vi "lv_icon.vi"(10 "Color icon in":T2, 11 "BW icon in":T2) -> (0 "Error code out":i32=43, 2 "Color icon out":T2, 3 "BW icon out":T2)   [LabVIEW 2021, in "lv_icon.lvlib"]
doc: "<p>Display this dialog box in one of the following ways:</p>\n\n<ul>\n<li>Double-click the <a href=\"nihelplauncher://docs/csh?context=lvcore_lvconcepts_using_icons\">icon</a> in the upper right corner of the front panel window, block diagram window, or <a href=\"nihelplauncher://docs/csh?context=lvcore_lvconcepts_custom_cont_ind_type\">Control Editor</a> window.</li>\n<li>Right-click the icon in the upper right corner of the front panel window, block diagram window, or <strong>Control Editor</strong> window and select <strong>Edit Icon</strong> from the shortcut menu.</li>\n<li>Select <strong>File<span class=\"U+187\">>></span>VI Properties</strong> or <strong>File<span class=\"U+187\">>></span>Control Properties</strong> to display the <a href=\"nihelplauncher://docs/csh?context=lvcore_lvdialog_vi_properties_dialog_box\">VI Properties</a> dialog box or <strong>Control Properties</strong> dialog box, respectively. Then select <strong>General</strong> from the <strong>Category</strong> pull-down menu and click the <strong>Edit Icon</strong> button.</li>\n<li>Right-click a project library, statechart, class, or XControl item in the <a href=\"nihelplauncher://docs/csh?context=lvcore_lvconcepts_using_labview_projects\">Project Explorer</a> window and select <strong> Properties</strong> from the shortcut menu to display the corresponding <strong>Properties</strong> dialog box. Then click the <strong>Edit</strong> button on the <strong>General Settings</strong> page.</li>\n</ul>\n\n<p>Use this dialog box to <a href=\"nihelplauncher://docs/csh?context=lvcore_lvhowto_creating_icons\">create and edit icons</a>.</p>"
uses:
  <vilib>/LabVIEW Icon API/lv_icon/lv_icon.lvlib
  <vilib>/LabVIEW Icon API/lv_icon/Controls/BodyText.ctl
  <vilib>/LabVIEW Icon API/lv_icon/Controls/Font.ctl
  <vilib>/LabVIEW Icon API/lv_icon/Controls/Alignment.ctl
  <vilib>/LabVIEW Icon API/lv_icon/Controls/Layer.ctl
  <resource>/plugins/NIIconEditor/Controls/LayerList.ctl
  <resource>/plugins/NIIconEditor/Controls/NewLayer.ctl
  <resource>/plugins/NIIconEditor/Controls/DeleteLayer.ctl
  <resource>/plugins/NIIconEditor/Controls/Arrow Up.ctl
  <resource>/plugins/NIIconEditor/Controls/Arrow Down.ctl
  <resource>/plugins/NIIconEditor/Controls/Framework Templates.ctl
  <vilib>/LabVIEW Icon API/lv_icon/Controls/Graphic.ctl
  <resource>/plugins/NIIconEditor/Controls/ColorChange.ctl
  <vilib>/LabVIEW Icon API/lv_icon/Controls/IEColor.ctl
  <resource>/plugins/NIIconEditor/Controls/Rotate.ctl
  <resource>/plugins/NIIconEditor/Controls/Flip.ctl
  <resource>/plugins/NIIconEditor/Controls/Tools.ctl
  <resource>/plugins/NIIconEditor/Controls/Pen.ctl
  <resource>/plugins/NIIconEditor/Controls/Line.ctl
  <resource>/plugins/NIIconEditor/Controls/Dropper.ctl
  <resource>/plugins/NIIconEditor/Controls/Fill.ctl
  <resource>/plugins/NIIconEditor/Controls/IERect.ctl
  <resource>/plugins/NIIconEditor/Controls/FRect.ctl
  <resource>/plugins/NIIconEditor/Controls/Circle.ctl
  <resource>/plugins/NIIconEditor/Controls/FCircle.ctl
  <resource>/plugins/NIIconEditor/Controls/Rubber.ctl
  <resource>/plugins/NIIconEditor/Controls/Text.ctl
  <resource>/plugins/NIIconEditor/Controls/Selection.ctl
  <resource>/plugins/NIIconEditor/Controls/Move.ctl
  <resource>/plugins/NIIconEditor/Controls/TextMarker.ctl
  <vilib>/picture/picture.llb/imagedata.ctl
  <resource>/plugins/NIIconEditor/Controls/Refresh.ctl
  <resource>/plugins/NIIconEditor/Controls/References Cluster.ctl
  <vilib>/Utility/miscctls.llb/LVPoint32TypeDef.ctl
  <vilib>/LabVIEW Icon API/lv_icon/Controls/Pathes.ctl
  <resource>/plugins/NIIconEditor/Controls/Path&Icon.ctl
  <resource>/plugins/NIIconEditor/Class/Ants/Ants.lvclass
  <resource>/plugins/NIIconEditor/Class/FakedArray/FakedArray.lvclass
  <vilib>/LabVIEW Icon API/lv_icon/Classes/Icon/Icon.lvclass
  <resource>/plugins/NIIconEditor/Class/Icon Library/Glyph.lvclass
  <resource>/dialog/lvconfig.llb/LV Config Read String.vi
  <resource>/dialog/lvconfig.llb/LV Config Write String.vi
panel:
  out "LabVIEW Icon out":string
  in  "LabVIEW Icon in":string
  out "Terminals":picture
  out "Preview2":picture
  out "TextMarker":T1="^"
  in  "Help":bool
  in  "Cancel":bool
  in  "OK":bool
  out "XYZ":string="X: 14\nY: 31\nZ: 1"
  out "RGB":string="R: 0\nG: 0\nB: 0"
  out "Icon":picture
  out "Clipboard":picture
  in  "Tab Control":T3(tab)
  in  "refreshTemplates":T4
  out "templates path str":string
  in  "Templates":string(tree)="<All>"
  in  "Filter templates by keyword":string
  in  "Framework Templates":T5={"Scrollbar"=0, "Path & Icon 1"={"Rectangle"={"left"=0, "top"=0, "right"=32, "bottom"=32}, "Path"=path "C:/Users/tsandris/Documents/LabVIEW Data/Icon Templates/VI/Frameworks/_blank.png", "Image"=bytes[0], "Filter"="VI\\Frameworks", "FileName"="_blank"}, "Path & Icon 2"={"Rectangle"={"left"=0, "top"=0, "right"=32, "bottom"=32}, "Path"=path "C:/Users/tsandris/Documents/LabVIEW Data/Icon Templates/Library/Frameworks/_blank.png", "Image"=bytes[0], "Filter"="Library\\Frameworks", "FileName"="_blank"}, "Path & Icon 3"={"Rectangle"={"left"=0, "top"=0, "right"=0, "bottom"=0}, "Path"=path "", "Image"=bytes[0], "Filter"="", "FileName"=""}, "Path & Icon 4"={"Rectangle"={"left"=0, "top"=0, "right"=0, "bottom"=0}, "Path"=path "", "Image"=bytes[0], "Filter"="", "FileName"=""}, "Path & Icon 5"={"Rectangle"={"left"=0, "top"=0, "right"=0, "bottom"=0}, "Path"=path "", "Image"=bytes[0], "Filter"="", "FileName"=""}, "Path & Icon 6"={"Rectangle"={"left"=0, "top"=0, "right"=0, "bottom"=0}, "Path"=path "", "Image"=bytes[0], "Filter"="", "FileName"=""}, "Path & Icon 7"={"Rectangle"={"left"=0, "top"=0, "right"=0, "bottom"=0}, "Path"=path "", "Image"=bytes[0], "Filter"="", "FileName"=""}, "Path & Icon 8"={"Rectangle"={"left"=0, "top"=0, "right"=0, "bottom"=0}, "Path"=path "", "Image"=bytes[0], "Filter"="", "FileName"=""}, "Path & Icon 9"={"Rectangle"={"left"=0, "top"=0, "right"=0, "bottom"=0}, "Path"=path "", "Image"=bytes[0], "Filter"="", "FileName"=""}, "Path & Icon 10"={"Rectangle"={"left"=0, "top"=0, "right"=0, "bottom"=0}, "Path"=path "", "Image"=bytes[0], "Filter"="", "FileName"=""}, "Path & Icon 11"={"Rectangle"={"left"=0, "top"=0, "right"=0, "bottom"=0}, "Path"=path "", "Image"=bytes[0], "Filter"="", "FileName"=""}, "Path & Icon 12"={"Rectangle"={"left"=0, "top"=0, "right"=0, "bottom"=0}, "Path"=path "", "Image"=bytes[0], "Filter"="", "FileName"=""}, "Path & Icon 13"={"Rectangle"={"left"=0, "top"=0, "right"=0, "bottom"=0}, "Path"=path "", "Image"=bytes[0], "Filter"="", "FileName"=""}, "Path & Icon 14"={"Rectangle"={"left"=0, "top"=0, "right"=0, "bottom"=0}, "Path"=path "", "Image"=bytes[0], "Filter"="", "FileName"=""}, "Path & Icon 15"={"Rectangle"={"left"=0, "top"=0, "right"=0, "bottom"=0}, "Path"=path "", "Image"=bytes[0], "Filter"="", "FileName"=""}, "Path & Icon 16"={"Rectangle"={"left"=0, "top"=0, "right"=0, "bottom"=0}, "Path"=path "", "Image"=bytes[0], "Filter"="", "FileName"=""}, "Path & Icon 17"={"Rectangle"={"left"=0, "top"=0, "right"=0, "bottom"=0}, "Path"=path "", "Image"=bytes[0], "Filter"="", "FileName"=""}, "Path & Icon 18"={"Rectangle"={"left"=0, "top"=0, "right"=0, "bottom"=0}, "Path"=path "", "Image"=bytes[0], "Filter"="", "FileName"=""}, "Path & Icon 19"={"Rectangle"={"left"=0, "top"=0, "right"=0, "bottom"=0}, "Path"=path "", "Image"=bytes[0], "Filter"="", "FileName"=""}, "Path & Icon 20"={"Rectangle"={"left"=0, "top"=0, "right"=0, "bottom"=0}, "Path"=path "", "Image"=bytes[0], "Filter"="", "FileName"=""}, "Path & Icon 21"={"Rectangle"={"left"=0, "top"=0, "right"=0, "bottom"=0}, "Path"=path "", "Image"=bytes[0], "Filter"="", "FileName"=""}, "Path & Icon 22"={"Rectangle"={"left"=0, "top"=0, "right"=0, "bottom"=0}, "Path"=path "", "Image"=bytes[0], "Filter"="", "FileName"=""}, "Path & Icon 23"={"Rectangle"={"left"=0, "top"=0, "right"=0, "bottom"=0}, "Path"=path "", "Image"=bytes[0], "Filter"="", "FileName"=""}, "Path & Icon 24"={"Rectangle"={"left"=0, "top"=0, "right"=0, "bottom"=0}, "Path"=path "", "Image"=bytes[0], "Filter"="", "FileName"=""}, "Path & Icon 25"={"Rectangle"={"left"=0, "top"=0, "right"=0, "bottom"=0}, "Path"=path "", "Image"=bytes[0], "Filter"="", "FileName"=""}, "Path & Icon 26"={"Rectangle"={"left"=0, "top"=0, "right"=0, "bottom"=0}, "Path"=path "", "Image"=bytes[0], "Filter"="", "FileName"=""}, "Path & Icon 27"={"Rectangle"={"left"=0, "top"=0, "right"=0, "bottom"=0}, "Path"=path "", "Image"=bytes[0], "Filter"="", "FileName"=""}, "Path & Icon 28"={"Rectangle"={"left"=0, "top"=0, "right"=0, "bottom"=0}, "Path"=path "", "Image"=bytes[0], "Filter"="", "FileName"=""}, "Path & Icon 29"={"Rectangle"={"left"=0, "top"=0, "right"=0, "bottom"=0}, "Path"=path "", "Image"=bytes[0], "Filter"="", "FileName"=""}, "Path & Icon 30"={"Rectangle"={"left"=0, "top"=0, "right"=0, "bottom"=0}, "Path"=path "", "Image"=bytes[0], "Filter"="", "FileName"=""}}
  in  "Body Text":T7={"Line 1 text"="", "Line 2 text"="", "Line 3 text"="", "Line 4 text"="", "Line 1 color"=0, "Line 2 color"=0, "Line 3 color"=0, "Line 4 color"=0, "Body Text Spec"={"Font"="", "Alignment"=1, "Size"=9}, "Center text vertically"=TRUE, "Capitalize Text"=TRUE} {"Body Text Spec"."Alignment" items=["left", "center", "right"]}
  in  "Filter glyphs by keyword":string
  in  "Glyphs":string(tree)="<All>"
  out "glyph path str":string
  out "Glyphs []":T6[][](array[typedef])
  in  "refreshGlyphs":T4
  in  "Add Layer":T10
  in  "Remove Layer":T11
  in  "Move Down":T12
  in  "Move Up":T13
  in  "Icon Template":T14={"LayerIcon"=bytes[0], "LayerName"="", "Opacity"=100, "Visibility?"=TRUE} {"Opacity" scale=0.0..100.0}
  in  "Icon Text":T14={"LayerIcon"=bytes[0], "LayerName"="Icon Text", "Opacity"=100, "Visibility?"=TRUE} {"Opacity" scale=0.0..100.0}
  in  "User Layers":T15={"Scrollbar"=0, "Layer 1"={"LayerIcon"=bytes[0], "LayerName"="VI Icon", "Opacity"=100, "Visibility?"=TRUE}, "Layer 2"={"LayerIcon"=bytes[3230], "LayerName"="", "Opacity"=100, "Visibility?"=TRUE}, "Layer 3"={"LayerIcon"=bytes[3230], "LayerName"="", "Opacity"=100, "Visibility?"=TRUE}, "Layer 4"={"LayerIcon"=bytes[3230], "LayerName"="", "Opacity"=100, "Visibility?"=TRUE}} {"Layer 4"."Opacity" scale=0.0..100.0; "Layer 3"."Opacity" scale=0.0..100.0; "Layer 2"."Opacity" scale=0.0..100.0; "Layer 1"."Opacity" scale=0.0..100.0}
  out "Preview":picture
  in  "Horizontal Flip":T16
  in  "Clockwise Rotate":T17
  in  "Swap":T18
  in  "Line Color":T19
  in  "Fill Color":T19=16777215
  in  "Tools":T20=enum."Rectangle"
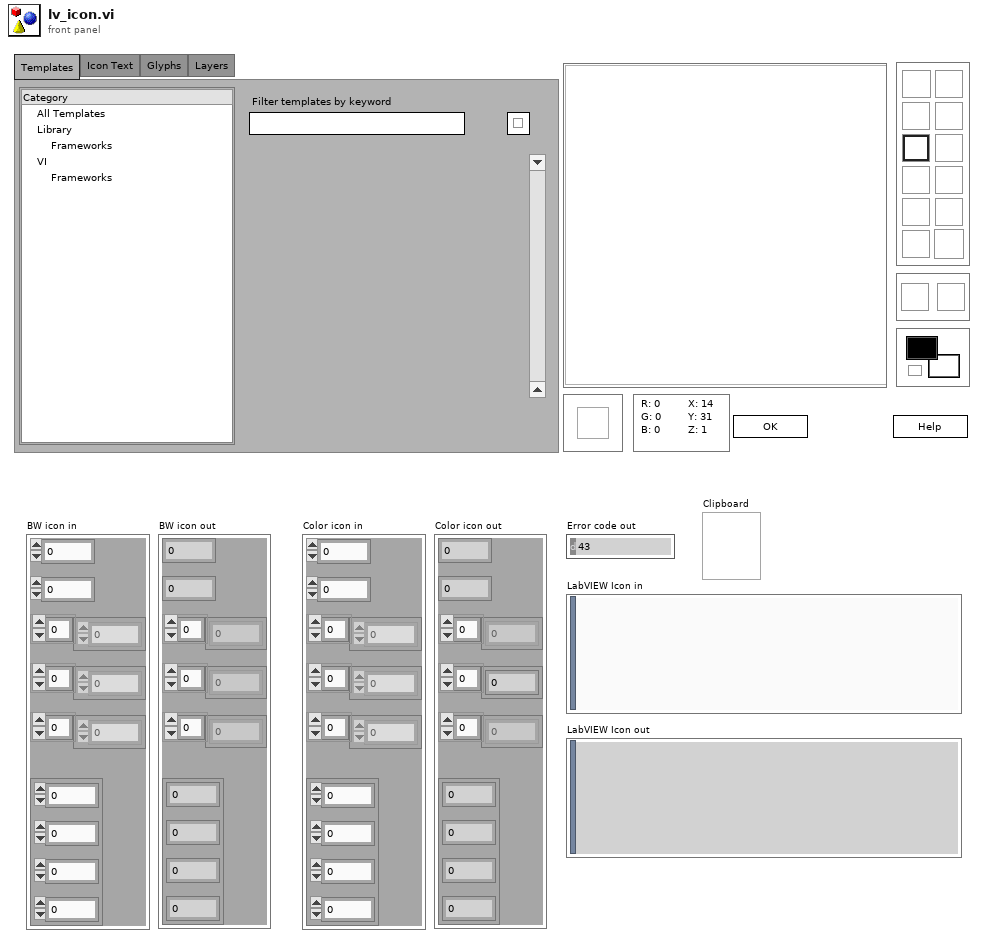
[diagram p1: front panel]
types:
  T1 = typedef "TextMarker.ctl" = string
  T2 = typedef "imagedata.ctl" = cluster{"image type":i32, "image depth":i32, "image":u8[], "mask":u8[], "colors":u32[], "Rectangle":cluster{"left":i16, "top":i16, "right":i16, "bottom":i16}}
  T3 = enum32{"Templates", "Icon Text", "Glyphs", "Layers"}
  T4 = typedef "Refresh.ctl" = bool
  T5 = typedef "Framework Templates.ctl" = cluster{"Scrollbar":i32, "Path & Icon 1":T6, "Path & Icon 2":T6, "Path & Icon 3":T6, "Path & Icon 4":T6, "Path & Icon 5":T6, "Path & Icon 6":T6, "Path & Icon 7":T6, "Path & Icon 8":T6, "Path & Icon 9":T6, "Path & Icon 10":T6, "Path & Icon 11":T6, "Path & Icon 12":T6, "Path & Icon 13":T6, "Path & Icon 14":T6, "Path & Icon 15":T6, "Path & Icon 16":T6, "Path & Icon 17":T6, "Path & Icon 18":T6, "Path & Icon 19":T6, "Path & Icon 20":T6, "Path & Icon 21":T6, "Path & Icon 22":T6, "Path & Icon 23":T6, "Path & Icon 24":T6, "Path & Icon 25":T6, "Path & Icon 26":T6, "Path & Icon 27":T6, "Path & Icon 28":T6, "Path & Icon 29":T6, "Path & Icon 30":T6}
  T6 = typedef "Graphic.ctl" = cluster{"Rectangle":cluster{"left":i16, "top":i16, "right":i16, "bottom":i16}, "Path":path, "Image":picture, "Filter":string, "FileName":string}
  T7 = typedef "BodyText.ctl" = cluster{"Line 1 text":string, "Line 2 text":string, "Line 3 text":string, "Line 4 text":string, "Line 1 color":u32, "Line 2 color":u32, "Line 3 color":u32, "Line 4 color":u32, "Body Text Spec":cluster{"Font":T8, "Alignment":T9, "Size":u8}, "Center text vertically":bool, "Capitalize Text":bool}
  T8 = typedef "Font.ctl" = string
  T9 = typedef "Alignment.ctl" = u16
  T10 = typedef "NewLayer.ctl" = bool
  T11 = typedef "DeleteLayer.ctl" = bool
  T12 = typedef "Arrow Down.ctl" = bool
  T13 = typedef "Arrow Up.ctl" = bool
  T14 = typedef "Layer.ctl" = cluster{"LayerIcon":picture, "LayerName":string, "Opacity":u8, "Visibility?":bool}
  T15 = typedef "LayerList.ctl" = cluster{"Scrollbar":i32, "Layer 1":T14, "Layer 2":T14, "Layer 3":T14, "Layer 4":T14}
  T16 = typedef "Flip.ctl" = bool
  T17 = typedef "Rotate.ctl" = bool
  T18 = typedef "ColorChange.ctl" = bool
  T19 = typedef "IEColor.ctl" = u32
  T20 = typedef "Tools.ctl" = enum32{"Pencil", "Line", "Dropper", "Fill", "Rectangle", "Filled Rectangle", "Ellipse", "Filled Ellipse", "Eraser", "Text", "Select", "Move"}
  T21 = enum32{"Invalid", "Standard", "Closed", "Hidden", "Minimized", "Maximized"}
  T22 = typedef "lv_icon.lvlib/References Cluster.ctl" = cluster{"Add Layer":refnum<vi>, "Remove Layer":refnum<vi>, "Line Text":refnum<vi>[], "Body Text Spec":refnum<vi>, "DNL_Font":refnum<vi>, "glyph path str":refnum<vi>, "templates path str":refnum<vi>, "Arrow Up":refnum<vi>, "Arrow Down":refnum<vi>, "IE VI Ref":refnum<vi>, "Glyphs tree":refnum<vi>, "Templates tree":refnum<vi>, "Layer Icon Text":refnum<vi>, "Layer Template":refnum<vi>, "Clipboard":refnum<vi>, "Body Text":refnum<vi>, "Search Templates":refnum<vi>, "TextMarker":refnum<vi>, "Tab Control":refnum<vi>, "Search Glyphs":refnum<vi>, "Line Color":refnum<vi>, "DNL_Glyphs []":refnum<vi>, "Fill Color":refnum<vi>, "Tools":refnum<vi>, "Icon":refnum<vi>, "Preview":refnum<vi>, "Ants":refnum<vi>, "Terminals":refnum<vi>, "menu reference":refnum<k9>, "LayerNames":refnum<vi>[], "GlyphLoadAnimation":refnum<vi>, "TemplateLoadAnimation":refnum<vi>, "refreshGlyphs":refnum<vi>, "refreshTemplates":refnum<vi>}
  T23 = cluster{"Left":i16, "Top":i16, "Right":i16, "Bottom":i16}
  T24 = typedef "LVAllMonitorsDisplayTypeDef.ctl" = cluster{"Bounds":cluster{"Left":i16, "Top":i16, "Right":i16, "Bottom":i16}, "Depth":i16}[]
  T25 = cluster{"Global stop?":refnum<user-event>, "Templates":refnum<user-event>, "Glyphs":refnum<user-event>}
  T26 = typedef "lv_icon.lvlib/Global Data.ctl" = cluster{"Class":T27, "Ref":T22, "Support":T28}
  T27 = typedef "IE Classes.ctl" = cluster{"Ants":refnum<class "Ants.lvclass">, "Layer":refnum<class "FakedArray.lvclass">, "Templates":refnum<class "FakedArray.lvclass">, "Icon":refnum<class "Icon.lvclass">, "Glyph":refnum<class "Glyph.lvclass">, "Settings":refnum<class "Settings.lvclass">, "Tools":refnum<class "Tools Paint.lvclass">}
  T28 = typedef "SupportClass.ctl" = cluster{"AntsRect":cluster{"left":i16, "top":i16, "right":i16, "bottom":i16}, "Mouse Move Coords":T29, "Mouse Down Coords":T29, "Temp Coord":T29, "Action":T30, "Edge Color":T19, "Fill Color":T19, "Mouse Down?":bool, "Draft Mode?":bool, "Temp Icon":picture, "CTRL Pressed":bool, "Move Selection?":bool, "AntsRect Orig":cluster{"left":i16, "top":i16, "right":i16, "bottom":i16}, "Text":string, "TM Set?":bool, "Mouse inside icon?":bool, "Tool (old value)":u32, "Pencil Move Color":u32, "Swap Colors?":bool, "Shift pressed?":bool}
  T29 = typedef "LVPoint32TypeDef.ctl" = cluster{"Horizontal":i32, "Vertical":i32}
  T30 = typedef "SupportClass_Action.ctl" = enum16{"Default", "Move Selection", "Glyph Library", "Tool"}
  T31 = typedef "Pathes.ctl" = enum16{"Root Path", "Icon Templates", "Icon Templates VI", "Icon Templates Lib", "Glyphs"}
  T32 = typedef "Path&Icon.ctl" = cluster{"Rectangle":cluster{"left":i16, "top":i16, "right":i16, "bottom":i16}, "Path":path, "Image":picture, "Filter":string, "FileName":string}
  T33 = typedef "lveventtype.ctl" = enum32{"Null", "Timeout", "Annotation Menu Selection", "Annotation Menu Selection?", "App Instance Close", "App Instance Close?", "Autoscale Range Change", "Bookmark Info Change", "Cell Edit", "Cell Edit?", "Cursor Grab", "Cursor Grab?", "Cursor Menu Selection", "Cursor Menu Selection?", "Cursor Move", "Cursor Release", "Data Change", "Direction Change", "Display State Change", "Drag Ended", "Drag Enter", "Drag Leave", "Drag Over", "Drag Source Update", "Drag Starting", "Drag Starting?", "Drop", "Exec State Change", "Key Down", "Key Down?", "Key Repeat", "Key Repeat?", "Key Up", "Listbox Double Click", "Menu Activation?", "Menu Selection (App)", "Menu Selection? (App)", "Menu Selection (User)", "Mouse Down", "Mouse Down?", "Mouse Enter", "Mouse Leave", "Mouse Move", "Mouse Up", "Mouse Wheel", "NI Security User Change (App)", "Pane Size", "Panel Close", "Panel Close?", "Panel Resize", "Plot Attribute Change", "Scale Range Change", "Shortcut Menu Activation?", "Shortcut Menu Selection (App)", "Shortcut Menu Selection? (App)", "Shortcut Menu Selection (User)", "Tree Double Click", "Tree Drag", "Tree Drag?", "Tree Drop", "Tree Drop?", "Tree Item Close", "Tree Item Close?", "Tree Item Open", "Tree Item Open?", "User Event", "Value Change"}
  T34 = typedef "eventvkey.ctl" = enum16{"ASCII", "Enter", "Return", "Shift", "Ctrl", "Alt", "Cmd", "Opt", "Caps", "NumLock", "Clear", "Break", "Up", "Down", "Left", "Right", "Insert", "Delete", "Home", "End", "PageUp", "PageDown", "Escape", "Help", "Pause", "ScrollLock", "F1", "F2", "F3", "F4", "F5", "F6", "F7", "F8", "F9", "F10", "F11", "F12", "F13", "F14", "F15", "F16", "F17", "F18", "F19", "F20", "F21", "F22", "F23", "F24", "Play", "VolumeUp", "VolumeDown", "Mute", "Two Byte Char"}
  T35 = cluster{"Shift":bool, "Ctrl":bool, "Alt":bool, "Cmd":bool, "Opt":bool}
  T36 = typedef "LVRectTypeDef.ctl" = cluster{"Left":i16, "Top":i16, "Right":i16, "Bottom":i16}
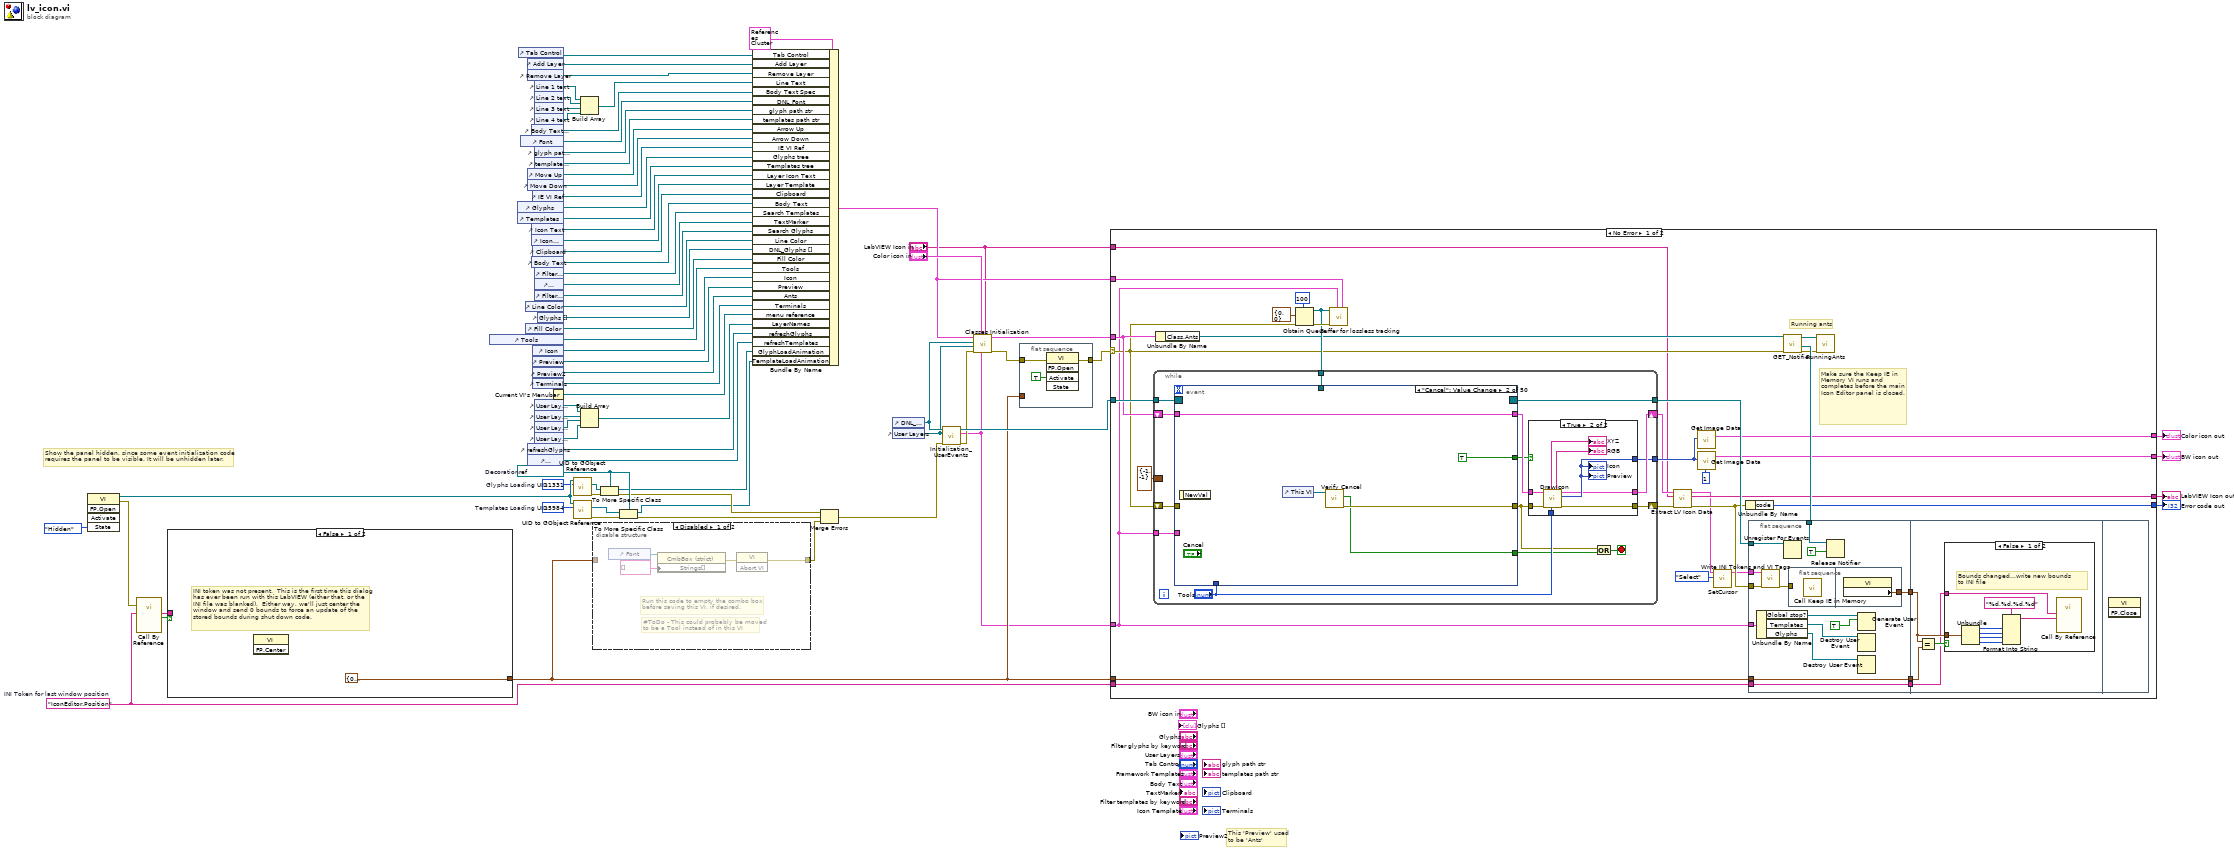
[diagram p0: block diagram]
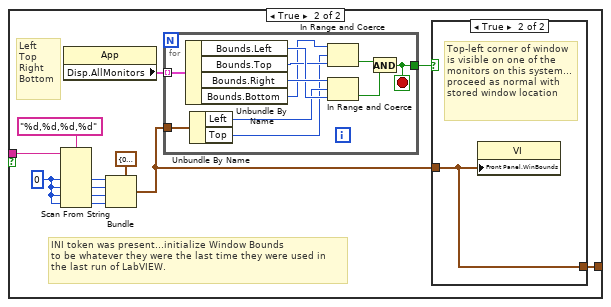
[diagram p2: hidden frame]
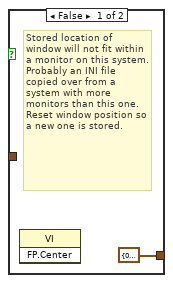
[diagram p3: hidden frame]
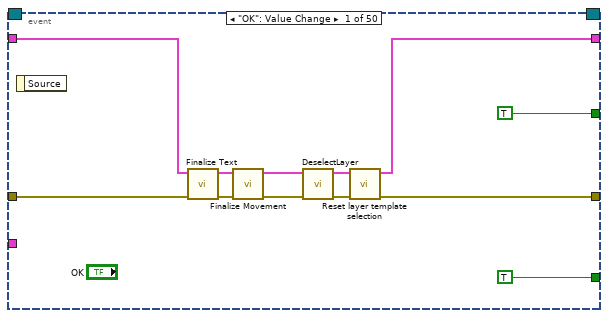
[diagram p6: hidden frame]
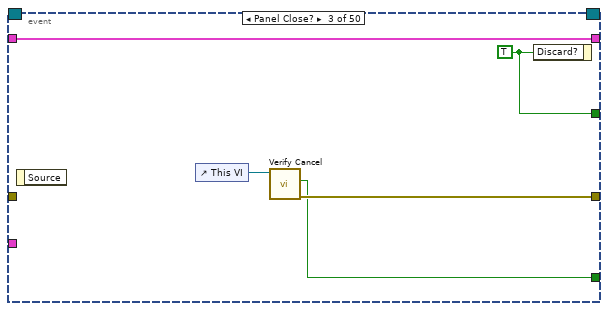
[diagram p7: hidden frame]
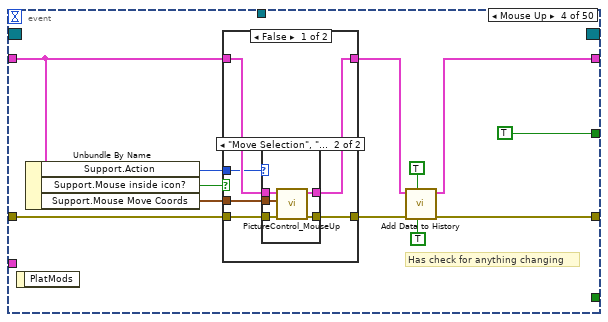
[diagram p8: hidden frame]
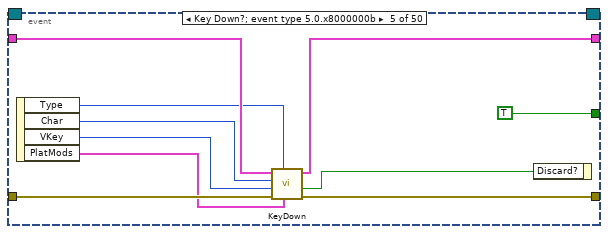
[diagram p11: hidden frame]
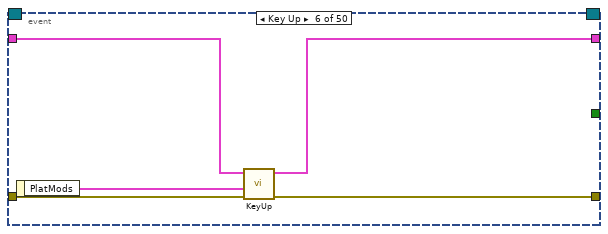
[diagram p12: hidden frame]
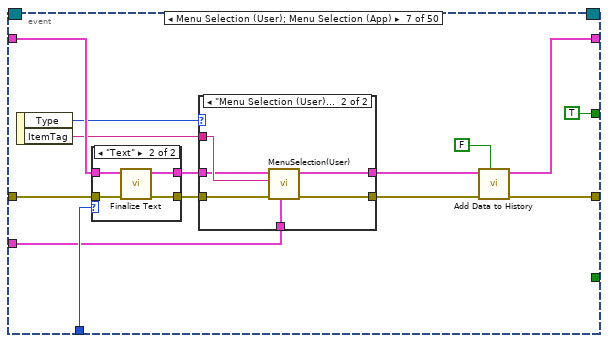
[diagram p13: hidden frame]
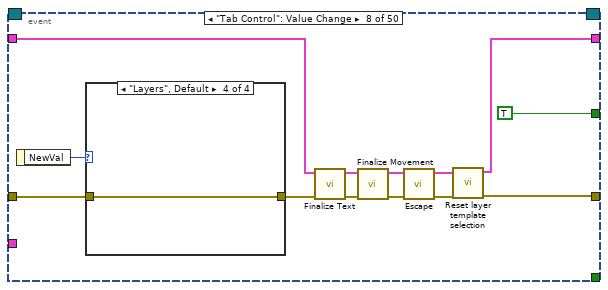
[diagram p16: hidden frame]
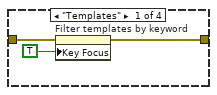
[diagram p17: hidden frame]
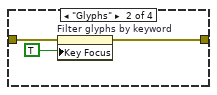
[diagram p18: hidden frame]
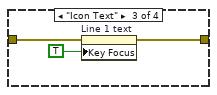
[diagram p19: hidden frame]
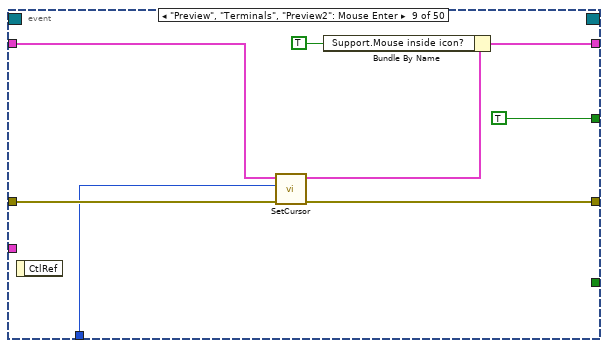
[diagram p20: hidden frame]
diagram:
  w13 = refnum<vi> refnum  # Decoration
  w11 = 15984  # Templates Loading UID
  w12 = 11331  # Glyphs Loading UID
  w24 = "IconEditor.Position"  # INI Token for last window position
  # "Show the panel hidden, since some event initialization code requires the panel to be visible. It will be unhidden later."
  # "This 'Preview' used\nto be 'Ants'"
  n1 = invoke class="VI" method="FP.Open"("State"=T21."Hidden") -> (reference out=w76:refnum<vi>, error out=w25:errorcluster)  [unwired: 4 in, 3 out]
  n2 = call-by-ref "?"(error in=w25, "key"=w24) -> ("found?"=w17:bool, "value"=w18:string)  [unwired: 5 in, 3 out]
  n3 = case shown="False" w17 {
    tunnel: [T23 {"Left"=0, "Top"=0, "Right"=0, "Bottom"=0} ("Front Panel.PanelBounds") w78] -> w19
    tunnel: w18 -> [_ w89]
    frame False {
      # "INI token was not present.  This is the first time this dialog\nhas ever been run with this LabVIEW (either that, or the\nINI file was blanked).  Either way, we'll just center the\nwindow and send 0 bounds to force an update of the\nstored bounds during shut down code."
      n4 = invoke class="VI" method="FP.Center"() -> ()  [unwired: 3 in, 3 out]
    }
    frame True {
      w87 = i16 0 ("default value 1")
      # "Left\nTop\nRight\nBottom"
      # "INI token was present...initialize Window Bounds\nto be whatever they were the last time they were used in\nthe last run of LabVIEW."
      n5 = Scan From String(format string="%d,%d,%d,%d", input string=w89, default 1=w87, default 2=w87, default 3=w87, default 4=w87) -> (output 1=w86:i16, output 2=w85:i16, output 3=w84:i16, output 4=w83:i16)  [unwired: 2 in, 3 out]
      n6 = property class="App"() -> ("Disp.AllMonitors"=w81:T24)  [unwired: 2 in, 2 out]
      n7 = Bundle(cluster=T23 {"Left"=0, "Top"=0, "Right"=0, "Bottom"=0} ("Front Panel.PanelBounds"), "Left"=w86, "Top"=w85, "Right"=w84, "Bottom"=w83) -> (w80:T23)
      n8 = for {
        tunnel: w81 -> [w102] mode=indexing
        tunnel: w80 -> [w101]
        tunnel: [w92] -> w79
        stop <- w92 stop-if-true
        n9 = Unbundle By Name(w102) -> ("Bounds.Left"=w99:i16, "Bounds.Top"=w97:i16, "Bounds.Right"=w100:i16, "Bounds.Bottom"=w96:i16)
        n10 = Unbundle By Name(w101) -> ("Left"=w98:i16, "Top"=w95:i16)
        n11 = In Range and Coerce(upper limit=w96, x=w95, lower limit=w97) -> (In Range?=w94:bool)  [unwired: 1 out]
        n12 = In Range and Coerce(upper limit=w100, x=w98, lower limit=w99) -> (In Range?=w93:bool)  [unwired: 1 out]
        n13 = And(x=w94, y=w93) -> (x .and. y?=w92:bool)
      }
      n14 = case shown="True" w79 {
        tunnel: w80 -> [_ w91]
        tunnel: [T23 {"Left"=0, "Top"=0, "Right"=0, "Bottom"=0} ("Front Panel.PanelBounds") w91] -> w78
        frame False {
          # "Stored location of window will not fit within a monitor on this system.  Probably an INI file copied over from a system with more monitors than this one.  Reset window position so a new one is stored."
          n15 = invoke class="VI" method="FP.Center"() -> ()  [unwired: 3 in, 3 out]
        }
        frame True {
          # "Top-left corner of window is visible on one of the monitors on this system... proceed as normal with stored window location"
          n16 = property class="VI"("Front Panel.WinBounds"=w91) -> ()  [unwired: 2 in, 2 out]
        }
      }
    }
  }
  n17 = control-ref of="Tools"() -> (w72:refnum<vi>)
  n18 = control-ref of="Glyphs"() -> (w55:refnum<vi>)
  n19 = control-ref of="Templates"() -> (w56:refnum<vi>)
  n20 = control-ref of="Tab Control"() -> (w22:refnum<vi>)
  n21 = control-ref of="Font"() -> (w37:refnum<vi>)
  n22 = control-ref of="Line Color"() -> (w70:refnum<vi>)
  n23 = control-ref of="Fill Color"() -> (w71:refnum<vi>)
  n24 = control-ref of="Add Layer"() -> (w40:refnum<vi>)
  n25 = control-ref of="Remove Layer"() -> (w41:refnum<vi>)
  n26 = control-ref of="Move Up"() -> (w52:refnum<vi>)
  n27 = control-ref of="Move Down"() -> (w53:refnum<vi>)
  n28 = control-ref of="refreshGlyphs"() -> (w27:refnum<vi>)
  n29 = control-ref of="refreshTemplates"() -> (w28:refnum<vi>)
  n30 = control-ref of="Body Text Spec"() -> (w49:refnum<vi>)
  n31 = control-ref of="Icon Text"() -> (w58:refnum<vi>)
  n32 = control-ref of="Icon Template"() -> (w59:refnum<vi>)
  n33 = control-ref of="Body Text"() -> (w65:refnum<vi>)
  n34 = control-ref of="IE VI Ref"() -> (w54:refnum<vi>)
  n35 = control-ref of="Clipboard"() -> (w61:refnum<vi>)
  n36 = control-ref of="Icon"() -> (w73:refnum<vi>)
  n37 = control-ref of="Preview"() -> (w74:refnum<vi>)
  n38 = control-ref of="Preview2"() -> (w48:refnum<vi>)
  n39 = control-ref of="Terminals"() -> (w64:refnum<vi>)
  n40 = control-ref of="Line 1 text"() -> (w43:refnum<vi>)
  n41 = control-ref of="Line 2 text"() -> (w44:refnum<vi>)
  n42 = control-ref of="Line 3 text"() -> (w45:refnum<vi>)
  n43 = control-ref of="Line 4 text"() -> (w46:refnum<vi>)
  n44 = control-ref of="glyph path str"() -> (w50:refnum<vi>)
  n45 = control-ref of="templates path str"() -> (w51:refnum<vi>)
  n46 = control-ref of="Filter templates by keyword"() -> (w67:refnum<vi>)
  n47 = control-ref of="TextMarker"() -> (w68:refnum<vi>)
  n48 = control-ref of="Filter glyphs by keyword"() -> (w69:refnum<vi>)
  n49 = control-ref of="User Layer 1"() -> (w32:refnum<vi>)
  n50 = control-ref of="User Layer 2"() -> (w33:refnum<vi>)
  n51 = control-ref of="User Layer 3"() -> (w34:refnum<vi>)
  n52 = control-ref of="User Layer 4"() -> (w35:refnum<vi>)
  n53 = control-ref of="Glyphs []"() -> (w38:refnum<vi>)
  n54 = Current VI's Menubar() -> (w63:refnum<k9>)
  n55 = call <vilib>:"UID to GObject Reference.vi"("UID"=w12, "Owning VI"=w76) -> ("error out"=w8:errorcluster, "GObject"=w10:refnum<vi>)  [unwired: 7 in, 1 out]
  n56 = call <vilib>:"UID to GObject Reference.vi"("UID"=w11, "Owning VI"=w76) -> ("error out"=w7:errorcluster, "GObject"=w9:refnum<vi>)  [unwired: 7 in, 1 out]
  n57 = Build Array(w43, w44, w45, w46) -> (w42:refnum<vi>[])
  n58 = Build Array(w32, w33, w34, w35) -> (w30:refnum<vi>[])
  n59 = disable-structure shown="Disabled" {
    disable-tunnel: [w103 _] -> w4
    disable-tunnel: w19 -> [_ _]
    frame Disabled {
      # "#ToDo - This could probably be moved\nto be a Tool instead of in this VI"
      # "Run this code to empty the combo box\nbefore saving this VI, if desired."
      n60 = control-ref of="Font"() -> (w106:refnum<vi>)
      n61 = property class="CmbBox (strict)"(reference=w106, "Strings[]"=string[] [] ("Strings []")) -> (error out=w104:errorcluster)  [unwired: 1 in, 1 out]
      n62 = invoke class="VI" method="Abort VI"(error in=w104) -> (error out=w103:errorcluster)  [unwired: 2 in, 2 out]
    }
    frame Enabled {
    }
  }
  n63 = To More Specific Class(target class=w13, reference=w10, error in=w8) -> (specific class reference=w2:refnum<vi>, error out=w6:errorcluster)
  n64 = To More Specific Class(target class=w13, reference=w9, error in=w7) -> (specific class reference=w1:refnum<vi>, error out=w5:errorcluster)
  n65 = Bundle By Name(cluster=T22 {"Add Layer"=refnum, "Remove Layer"=refnum, "Line Text"=[], "Body Text Spec"=refnum, "DNL_Font"=refnum, "glyph path str"=refnum, "templates path str"=refnum, "Arrow Up"=refnum, "Arrow Down"=refnum, "IE VI Ref"=refnum, "Glyphs tree"=refnum, "Templates tree"=refnum, "Layer Icon Text"=refnum, "Layer Template"=refnum, "Clipboard"=refnum, "Body Text"=refnum, "Search Templates"=refnum, "TextMarker"=refnum, "Tab Control"=refnum, "Search Glyphs"=refnum, "Line Color"=refnum, "DNL_Glyphs []"=refnum, "Fill Color"=refnum, "Tools"=refnum, "Icon"=refnum, "Preview"=refnum, "Ants"=refnum, "Terminals"=refnum, "menu reference"=refnum, "LayerNames"=[], "GlyphLoadAnimation"=refnum, "TemplateLoadAnimation"=refnum, "refreshGlyphs"=refnum, "refreshTemplates"=refnum} ("references"), "Tab Control"=w22, "Add Layer"=w40, "Remove Layer"=w41, "Line Text"=w42, "Body Text Spec"=w49, "DNL_Font"=w37, "glyph path str"=w50, "templates path str"=w51, "Arrow Up"=w52, "Arrow Down"=w53, "IE VI Ref"=w54, "Glyphs tree"=w55, "Templates tree"=w56, "Layer Icon Text"=w58, "Layer Template"=w59, "Clipboard"=w61, "Body Text"=w65, "Search Templates"=w67, "TextMarker"=w68, "Search Glyphs"=w69, "Line Color"=w70, "DNL_Glyphs []"=w38, "Fill Color"=w71, "Tools"=w72, "Icon"=w73, "Preview"=w74, "Ants"=w48, "Terminals"=w64, "menu reference"=w63, "LayerNames"=w30, "refreshGlyphs"=w27, "refreshTemplates"=w28, "GlyphLoadAnimation"=w2, "TemplateLoadAnimation"=w1) -> (w31:T22)
  n66 = Merge Errors(w6, w5, w4) -> (w3:errorcluster)
  n67 = control-ref of="DNL_Framework Templates"() -> (w15:refnum<vi>)
  n68 = control-ref of="User Layers"() -> (w14:refnum<vi>)
  n69 = call <resource>:"Initialization_UserEvents.vi"("error in"=w3, "Layer Clusters"=w14, "DNL_Framework Templates"=w15) -> ("error out"=w60:errorcluster, "User events"=w16:T25, "Events"=w66:refnum<event-registration>)  [unwired: 6 out]
  n70 = call <resource>:"Classes Initialization.vi"("LabVIEW Icon in"="LabVIEW Icon in", "User events"=w16, "Color icon in"="Color icon in", "error in"=w60, "Layer Clusters"=w14, "DNL_Framework Templates"=w15, "Ref Cluster"=w31) -> ("error out"=w21:errorcluster, "Data out"=w47:T26)  [unwired: 3 out]
  n71 = flat-sequence {
    tunnel: w21 -> [w108]
    tunnel: w19 -> [_]
    tunnel: [w107] -> w20
    frame #0 {
      n72 = invoke class="VI" method="FP.Open"(error in=w108, "Activate"=TRUE ("Activate?")) -> (error out=w107:errorcluster)  [unwired: 3 in, 4 out]
    }
  }
  n73 = case shown="No Error" w20 {
    selector: w20 -> [w124 w828]
    tunnel: w66 -> [w141 _]
    tunnel: [w139 w829] -> w62
    tunnel: [w136 _] -> w57
    tunnel: w16 -> [w110 _]
    tunnel: w47 -> [w129 _]
    tunnel: w31 -> [w127 _]
    tunnel: [w126 _] -> w39
    tunnel: "LabVIEW Icon in" -> [w119 w827]
    tunnel: [w122 w827] -> w36
    tunnel: w19 -> [w115 _]
    tunnel: w24 -> [w111 _]
    frame No Error {
      # "Make sure the Keep IE in Memory VI runs and completes before the main Icon Editor panel is closed."
      # "Running ants"
      n74 = Unbundle By Name(w129) -> ("Class.Ants"=w128:refnum<class "Ants.lvclass">)
      n75 = Obtain Queue(max queue size (-1, unlimited)=100, element data type=T29 {"Horizontal"=0, "Vertical"=0} ("Coords"), error in (no error)=w124) -> (queue out=w130:refnum<queue>, error out=w131:errorcluster)  [unwired: 1 in, 2 out]
      n76 = while {
        shift-right: [w147] -> w121
        shift-left: w124 -> [w154]
        tunnel: [w151] -> w142
        tunnel: w141 -> [w150]
        tunnel: [w149] -> w138
        tunnel: w130 -> [w145]
        shift-right: [w156] -> w123
        shift-left: w129 -> [w144]
        border: T29 {"Horizontal"=-1, "Vertical"=-1} ("Corrected Out") -> [_]
        tunnel: w110 -> [w143]
        stop <- w152 stop-if-true
        n77 = event shown="[1] \"Cancel\": Value Change" {
          selector: w150 -> [_ _ _ _ _ _ _ _ _ _ _ _ _ _ _ _ _ _ _ _ _ _ _ _ _ _ _ _ _ _ _ _ _ _ _ _ _ _ _ _ _ _ _ _ _ _ _ _ _ _]
          dyn-events: [_ _ _ _ _ _ _ _ _ _ _ _ _ _ _ _ _ _ _ _ _ _ _ _ _ _ _ _ _ _ _ _ _ _ _ _ _ _ _ _ _ _ _ _ _ _ _ _ _ _] -> w151
          timeout: _ -> [_ _ _ _ _ _ _ _ _ _ _ _ _ _ _ _ _ _ _ _ _ _ _ _ _ _ _ _ _ _ _ _ _ _ _ _ _ _ _ _ _ _ _ _ _ _ _ _ _ _]
          tunnel: [w173 w183 w188 w193 w225 w231 w234 w268 w289 w299 w312 w329 w333 w339 w343 w356 w368 w382 w397 w408 w433 w440 w451 w467 w488 w496 w514 w534 w539 w543 w550 w561 w581 w596 w611 w622 w635 w651 w660 w669 w692 w705 w720 w730 w732 w751 w768 w788 w795 w797] -> w148
          tunnel: w154 -> [w175 _ _ w199 w226 w230 w242 w270 w290 w300 w312 w330 w336 w341 w348 w360 w367 w376 w399 w417 w434 w443 w456 w469 w491 w510 w522 w535 w540 w544 w551 w573 w586 w599 w615 w623 w641 w655 w661 w672 w695 w713 w723 w729 w741 w758 w772 w789 w795 w798]
          tunnel: [TRUE w182 w187 _ _ _ _ _ _ _ _ _ _ _ _ _ _ _ _ _ _ _ _ _ _ _ _ _ _ _ _ _ _ _ _ _ _ _ _ _ _ _ _ _ _ _ _ _ _ _] -> w153
          tunnel: "Tools" -> [_ _ _ _ _ _ w240 _ w288 _ _ _ _ _ _ _ _ _ _ _ _ _ _ _ _ _ _ _ _ _ _ _ _ _ _ _ _ _ _ _ _ _ _ _ _ _ _ _ _ _]
          tunnel: [TRUE TRUE ("Yes") w186 TRUE ("Yes") TRUE _ TRUE TRUE TRUE TRUE _ TRUE TRUE _ TRUE TRUE TRUE TRUE TRUE TRUE _ _ TRUE TRUE _ _ _ _ _ _ TRUE TRUE TRUE _ TRUE _ TRUE _ _ TRUE TRUE _ _ _ _ _ TRUE _ _ _] -> w146
          tunnel: w145 -> [_ _ _ _ _ _ _ _ _ w297 _ _ _ _ _ _ _ _ _ _ _ _ _ _ _ _ _ _ _ _ _ _ _ _ _ _ _ _ _ _ _ _ _ _ _ _ _ _ _ _]
          tunnel: w144 -> [w172 w184 w189 w198 w221 w229 w245 w266 w286 w296 w309 w326 w332 w338 w347 w359 w366 w378 w392 w404 w437 w439 w447 w465 w484 w501 w519 w532 w542 w546 w548 w569 w577 w594 w607 w620 w633 w657 w658 w679 w690 w703 w719 w727 w737 w756 w765 w786 w794 w799]
          tunnel: [w168 w184 w189 w191 w218 w227 w236 w260 w284 w295 w311 w325 w331 w337 w352 w354 w364 w381 w393 w409 w422 w438 w445 w463 w483 w494 w515 w532 w542 w545 w547 w562 w575 w593 w606 w619 w632 w649 w659 w665 w689 w707 w718 w725 w733 w750 w762 w786 w794 w799] -> w157
          tunnel: w143 -> [_ _ _ _ _ _ w232 _ _ _ _ _ _ _ _ _ _ _ _ _ _ _ _ _ _ _ _ w533 _ _ _ _ _ _ _ _ _ _ _ _ _ _ _ _ _ _ _ w787 _ _]
          event "OK": Value Change {
            n78 = event-data() -> ()  [unwired: 2 out]
            n79 = call <resource>:"Finalize Text.vi"("error in (no error)"=w175, "Data in"=w172) -> ("error out"=w176:errorcluster, "Data out"=w171:T26)  [unwired: 8 out]
            n80 = call <resource>:"Finalize Movement.vi"("error in (no error)"=w176, "Data in"=w171) -> ("error out"=w177:errorcluster, "Data out"=w170:T26)  [unwired: 1 in, 7 out]
            n81 = call <resource>:"DeselectLayer.vi"("error in (no error)"=w177, "Data in"=w170) -> ("error out"=w174:errorcluster, "Data out"=w169:T26)  [unwired: 8 out]
            n82 = call <resource>:"Reset layer template selection.vi"("error in (no error)"=w174, "Data in"=w169) -> ("error out"=w173:errorcluster, "Data out"=w168:T26)  [unwired: 1 in, 7 out]
          }
          event "Cancel": Value Change {
            n83 = event-data() -> ()  [unwired: 2 out]
            n84 = control-ref of="This VI"() -> (w180:refnum<vi>)
            n85 = call <resource>:"Verify Cancel.vi"("Calling VI"=w180) -> ("error out"=w183:errorcluster, "Close IE"=w182:bool)  [unwired: 9 in]
          }
          event Panel Close? {
            w186 = TRUE ("Discard?")
            n86 = event-data() -> ()  [unwired: 2 out]
            n87 = control-ref of="This VI"() -> (w185:refnum<vi>)
            n88 = call <resource>:"Verify Cancel.vi"("Calling VI"=w185) -> ("error out"=w188:errorcluster, "Close IE"=w187:bool)  [unwired: 9 in]
            n89 = event-data("Discard?"=w186) -> ()  [unwired: 1 in, 1 out]
          }
          event Mouse Up {
            # "Has check for anything changing"
            n90 = event-data() -> ()  [unwired: 2 out]
            n91 = Unbundle By Name(w198) -> ("Support.Action"=w196:T30, "Support.Mouse inside icon?"=w201:bool, "Support.Mouse Move Coords"=w197:T29)
            n92 = case shown="False" w201 {
              tunnel: w199 -> [w205 w216]
              tunnel: [w203 w216] -> w194
              tunnel: [w206 w215] -> w192
              tunnel: w198 -> [w207 w215]
              tunnel: w197 -> [w204 _]
              tunnel: w196 -> [w202 _]
              frame False {
                n93 = case shown="\"Move Selection\", \"Tool\"" w202 {
                  tunnel: w207 -> [w209 w214]
                  tunnel: [w209 w213] -> w206
                  tunnel: w205 -> [w208 w212]
                  tunnel: w204 -> [_ w211]
                  tunnel: [w208 w210] -> w203
                  frame "Default", Default {
                  }
                  frame "Move Selection", "Tool" {
                    n94 = call <resource>:"PictureControl_MouseUp.vi"("error in"=w212, "Coords"=w211, "Data in"=w214) -> ("error out"=w210:errorcluster, "Data out"=w213:T26)  [unwired: 4 in, 3 out]
                  }
                }
              }
              frame True {
              }
            }
            n95 = call <resource>:"Add Data to History.vi"("Check special fields? (F)"=TRUE, "Add to Undo?"=TRUE, "error in"=w194, "Data in"=w192) -> ("error out"=w193:errorcluster, "Data out"=w191:T26)  [unwired: 6 out]
          }
          event Key Down?; event type 5.0.x8000000b {
            n96 = event-data() -> ("Type"=w220:T33, "Char"=w217:i16, "VKey"=w224:T34, "PlatMods"=w219:T35)  [unwired: 1 out]
            n97 = call <resource>:"KeyDown.vi"("PlatMods"=w219, "Type"=w220, "error in (no error)"=w226, "VKey"=w224, "Char"=w217, "Data in"=w221) -> ("error out"=w225:errorcluster, "Discard?"=w223:bool, "Data out"=w218:T26)  [unwired: 3 out]
            n98 = event-data("Discard?"=w223) -> ()  [unwired: 1 in, 1 out]
          }
          event Key Up {
            n99 = event-data() -> ("PlatMods"=w228:T35)  [unwired: 1 out]
            n100 = call <resource>:"KeyUp.vi"("error in (no error)"=w230, "PlatMods"=w228, "Data in"=w229) -> ("error out"=w231:errorcluster, "Data out"=w227:T26)  [unwired: 7 out]
          }
          event Menu Selection (User); Menu Selection (App) {
            n101 = event-data() -> ("Type"=w243:T33, "ItemTag"=w244:string)  [unwired: 1 out]
            n102 = case shown="\"Text\"" w240 {
              tunnel: w242 -> [w246 w251]
              tunnel: w245 -> [w247 w250]
              tunnel: [w246 w249] -> w238
              tunnel: [w247 w248] -> w239
              frame Default {
              }
              frame "Text" {
                n103 = call <resource>:"Finalize Text.vi"("error in (no error)"=w251, "Data in"=w250) -> ("error out"=w249:errorcluster, "Data out"=w248:T26)  [unwired: 8 out]
              }
            }
            n104 = case shown="\"Menu Selection (User)\"" w243 {
              tunnel: w244 -> [_ w259]
              tunnel: [w253 w258] -> w235
              tunnel: w238 -> [w253 w257]
              tunnel: w232 -> [_ w256]
              tunnel: w239 -> [w252 w255]
              tunnel: [w252 w254] -> w237
              frame Default {
              }
              frame "Menu Selection (User)" {
                n105 = call <resource>:"MenuSelection(User).vi"("User events"=w256, "error in"=w257, "ItemTag"=w259, "Data in"=w255) -> ("error out"=w258:errorcluster, "Data out"=w254:T26)  [unwired: 1 in, 5 out]
              }
            }
            n106 = call <resource>:"Add Data to History.vi"("Add to Undo?"=FALSE, "error in"=w235, "Data in"=w237) -> ("error out"=w234:errorcluster, "Data out"=w236:T26)  [unwired: 7 in]
          }
          event "Tab Control": Value Change {
            n107 = event-data() -> ("NewVal"=w271:T3)  [unwired: 1 out]
            n108 = case shown="\"Layers\", Default" w271 {
              tunnel: w270 -> [w275 w278 w280 w282]
              tunnel: [w274 w277 w281 w282] -> w269
              frame "Templates" {
                n109 = property on="Filter templates by keyword" class="Str"(error in=w275, "Key Focus"=TRUE) -> (error out=w274:errorcluster)  [unwired: 1 in, 1 out]
              }
              frame "Glyphs" {
                n110 = property on="Filter glyphs by keyword" class="Str"(error in=w278, "Key Focus"=TRUE) -> (error out=w277:errorcluster)  [unwired: 1 in, 1 out]
              }
              frame "Icon Text" {
                n111 = property on="Line 1 text" class="Str"(error in=w280, "Key Focus"=TRUE) -> (error out=w281:errorcluster)  [unwired: 1 in, 1 out]
              }
              frame "Layers", Default {
              }
            }
            n112 = call <resource>:"Finalize Text.vi"("error in (no error)"=w269, "Data in"=w266) -> ("error out"=w272:errorcluster, "Data out"=w265:T26)  [unwired: 8 out]
            n113 = call <resource>:"Finalize Movement.vi"("error in (no error)"=w272, "Data in"=w265) -> ("error out"=w264:errorcluster, "Data out"=w262:T26)  [unwired: 1 in, 7 out]
            n114 = call <resource>:"Escape.vi"("error in"=w264, "Data in"=w262) -> ("error out"=w263:errorcluster, "Data out"=w261:T26)  [unwired: 1 in, 7 out]
            n115 = call <resource>:"Reset layer template selection.vi"("error in (no error)"=w263, "Data in"=w261) -> ("error out"=w268:errorcluster, "Data out"=w260:T26)  [unwired: 1 in, 7 out]
          }
          event "Preview", "Terminals", "Preview2": Mouse Enter {
            n116 = event-data() -> ()  [unwired: 2 out]
            n117 = call <resource>:"SetCursor.vi"("error in (no error)"=w290, "Radio Buttons"=w288, "Data in"=w286) -> ("error out"=w289:errorcluster, "Data out"=w285:T26)  [unwired: 7 out]
            n118 = Bundle By Name(cluster=w285, "Support.Mouse inside icon?"=TRUE) -> (w284:T26)
          }
          event "Preview", "Terminals", "Preview2": Mouse Move {
            n119 = event-data() -> ("Coords"=w294:T29)  [unwired: 1 out]
            n120 = call <resource>:"CoordinatesCorrection.vi"("Coordinates In"=w294) -> ("Corrected Out"=w291:T29)  [unwired: 10 out]
            n121 = feedback-in #1(w291) -> ()
            n122 = feedback #1() -> (w293:T29)
            n123 = Not Equal?(x=w293, y=w291) -> (x != y?=w292:bool)
            n124 = case shown="True" w292 {
              tunnel: w300 -> [w302 w308]
              tunnel: [w302 w307] -> w299
              tunnel: w297 -> [_ w306]
              tunnel: w296 -> [w301 w305]
              tunnel: [w301 w304] -> w295
              tunnel: w291 -> [_ w303]
              frame False {
              }
              frame True {
                n125 = call <resource>:"MouseMove.vi"("Buffer"=w306, "error in"=w308, "Coords"=w303, "Data in"=w305) -> ("error out"=w307:errorcluster, "Data out"=w304:T26)  [unwired: 6 out]
              }
            }
          }
          event "Preview", "Preview2", "Terminals": Mouse Leave {
            n126 = event-data() -> ()  [unwired: 2 out]
            n127 = Bundle By Name(cluster=w309, "Support.Mouse inside icon?"=FALSE) -> (w311:T26)
          }
          event "Preview", "Terminals", "Preview2": Mouse Down {
            # "Left click"
            n128 = event-data() -> ("Button"=w315:u16, "Coords"=w328:T29)  [unwired: 1 out]
            n129 = Not Equal?(x=u16 1, y=w315) -> (x != y?=w313:bool)
            n130 = control-ref of="This VI"() -> (w324:refnum<vi>)
            n131 = call <resource>:"Defer_FP_Updates.vi"("Defer Panel Updates"=TRUE, "error in (no error)"=w330, "lv_icon.vi in"=w324) -> ("error out"=w320:errorcluster, "lv icon.vi out"=w322:refnum<vi>)  [unwired: 7 out]
            n132 = call <resource>:"Reset layer template selection.vi"("Force reset? (T)"=FALSE, "error in (no error)"=w320, "Data in"=w326) -> ("error out"=w319:errorcluster, "Data out"=w316:T26)  [unwired: 1 in, 6 out]
            n133 = call <resource>:"MouseDown.vi"("Flip colors?"=w313, "error in"=w319, "Coords"=w328, "Data in"=w316) -> ("error out"=w318:errorcluster, "Data out"=w325:T26)  [unwired: 1 in, 5 out]
            n134 = call <resource>:"Defer_FP_Updates.vi"("Defer Panel Updates"=FALSE, "error in (no error)"=w318, "lv_icon.vi in"=w322) -> ("error out"=w329:errorcluster)  [unwired: 8 out]
          }
          event "Preview", "Terminals", "Preview2": Mouse Up {
            n135 = event-data() -> ("Coords"=w335:T29)  [unwired: 1 out]
            n136 = call <resource>:"PictureControl_MouseUp.vi"("error in"=w336, "Coords"=w335, "Data in"=w332) -> ("error out"=w333:errorcluster, "Data out"=w331:T26)  [unwired: 4 in, 3 out]
          }
          event Value Change {
            n137 = event-data() -> ("NewVal"=w340:T20)  [unwired: 1 out]
            n138 = call <resource>:"Value Change_Tools.vi"("error in"=w341, "NewVal"=w340, "Data in"=w338) -> ("error out"=w339:errorcluster, "Data out"=w337:T26)  [unwired: 7 out]
          }
          event Mouse Down {
            n139 = event-data() -> ("Mods.Double Click"=w342:bool)  [unwired: 1 out]
            n140 = call <resource>:"Finalize Text.vi"("error in (no error)"=w348, "Data in"=w347) -> ("error out"=w350:errorcluster, "Data out"=w349:T26)  [unwired: 8 out]
            n141 = call <resource>:"Finalize Movement.vi"("error in (no error)"=w350, "Data in"=w349) -> ("error out"=w346:errorcluster, "Data out"=w345:T26)  [unwired: 1 in, 7 out]
            n142 = call <resource>:"Mouse Down.vi"("error in"=w346, "Double Click"=w342, "Data in"=w345) -> ("error out"=w343:errorcluster, "Data out"=w344:T26)  [unwired: 7 out]
            n143 = Bundle By Name(cluster=w344, "Support.Tool (old value)"=u32 111) -> (w352:T26)
          }
          event Mouse Down {
            n144 = event-data() -> ()  [unwired: 2 out]
            n145 = call <resource>:"Finalize Text.vi"("error in (no error)"=w360, "Data in"=w359) -> ("error out"=w361:errorcluster, "Data out"=w358:T26)  [unwired: 8 out]
            n146 = call <resource>:"Finalize Movement.vi"("error in (no error)"=w361, "Data in"=w358) -> ("error out"=w357:errorcluster, "Data out"=w355:T26)  [unwired: 1 in, 7 out]
            n147 = call <resource>:"Escape.vi"("error in"=w357, "Data in"=w355) -> ("error out"=w356:errorcluster, "Data out"=w354:T26)  [unwired: 1 in, 7 out]
          }
          event Value Change {
            n148 = event-data() -> ()  [unwired: 2 out]
            n149 = call <vilib>:"Check Color.vi"("Color in"="Fill Color") -> ("Color out"=w369:T19)  [unwired: 26 out]
            n150 = call <vilib>:"Check Color.vi"("Color in"="Line Color") -> ("Color out"=w370:T19)  [unwired: 26 out]
            n151 = Bundle By Name(cluster=w366, "Support.Fill Color"=w369, "Support.Edge Color"=w370) -> (w365:T26)
            n152 = call <resource>:"Escape.vi"("Reset cursor (T)"=FALSE ("Reset cursor? (T)"), "error in"=w367, "Data in"=w365) -> ("error out"=w368:errorcluster, "Data out"=w364:T26)  [unwired: 1 in, 6 out]
          }
          event Value Change {
            n153 = event-data() -> ()  [unwired: 2 out]
            n154 = call <resource>:"Finalize Text.vi"("error in (no error)"=w376, "Data in"=w378) -> ("error out"=w380:errorcluster, "Data out"=w379:T26)  [unwired: 8 out]
            n155 = local read "Line Color"() -> (w375:T19)
            n156 = local read "Fill Color"() -> (w385:T19)
            n157 = call <resource>:"Finalize Movement.vi"("error in (no error)"=w380, "Data in"=w379) -> ("error out"=w374:errorcluster, "Data out"=w377:T26)  [unwired: 1 in, 7 out]
            n158 = stacked-sequence {
              tunnel: w385 -> [w389]
              tunnel: [w388] -> w383
              tunnel: w375 -> [w387]
              tunnel: w374 -> [w386]
              frame #0 {
                n159 = local write "Fill Color"(w387) -> ()
                n160 = property on="Line Color" class="ColBox (strict)"(error in=w386, "Val(Sgnl)"=w389) -> (error out=w388:errorcluster)  [unwired: 1 in, 1 out]
              }
            }
            n161 = call <resource>:"Escape.vi"("error in"=w383, "Data in"=w377) -> ("error out"=w382:errorcluster, "Data out"=w381:T26)  [unwired: 1 in, 7 out]
          }
          event Value Change {
            n162 = event-data() -> ()  [unwired: 2 out]
            n163 = call <resource>:"Finalize Text.vi"("error in (no error)"=w399, "Data in"=w392) -> ("error out"=w398:errorcluster, "Data out"=w394:T26)  [unwired: 8 out]
            n164 = call <resource>:"Finalize Movement.vi"("error in (no error)"=w398, "Data in"=w394) -> ("error out"=w395:errorcluster, "Data out"=w391:T26)  [unwired: 1 in, 7 out]
            n165 = call <resource>:"RotateFlip.vi"("error in"=w395, "Rotate"="Clockwise Rotate", "Data in"=w391) -> ("error out"=w396:errorcluster, "Data out"=w390:T26)  [unwired: 2 in, 5 out]
            n166 = call <resource>:"Escape.vi"("error in"=w396, "Data in"=w390) -> ("error out"=w397:errorcluster, "Data out"=w393:T26)  [unwired: 1 in, 7 out]
          }
          event User Event {
            # "This is an initialization event for the templates"
            n167 = event-data() -> ("Templates"=w419:string)  [unwired: 1 out]
            n168 = Unbundle By Name(w404) -> ("Ref.TemplateLoadAnimation"=w403:refnum<vi>, "Ref.refreshTemplates"=w402:refnum<vi>)
            n169 = control-ref of="This VI"() -> (w414:refnum<vi>)
            n170 = call <resource>:"Defer_FP_Updates.vi"("Defer Panel Updates"=TRUE, "error in (no error)"=w417, "lv_icon.vi in"=w414) -> ("error out"=w412:errorcluster, "lv icon.vi out"=w411:refnum<vi>)  [unwired: 7 out]
            n171 = Unflatten From String(type=cluster{T6[], i32, bool} {[], 0, FALSE}, binary string=w419, error in (no error)=w412) -> (value=w410:cluster{T6[], i32, bool}, error out=w415:errorcluster)  [unwired: 3 out]
            n172 = call <resource>:"Process Template Graphics.vi"("error in (no error)"=w415, "Data"=w410, "Data in"=w404) -> ("error out"=w407:errorcluster, "Data out"=w409:T26)  [unwired: 7 out]
            n173 = call <resource>:"ChangeRefreshGraphicsState.vi"("error in (no error)"=w407, "refreshing?"=FALSE, "button ref"=w402, "animatedDecoration ref"=w403) -> ("error out"=w406:errorcluster)  [unwired: 7 in]
            n174 = call <resource>:"Defer_FP_Updates.vi"("error in (no error)"=w406, "lv_icon.vi in"=w411) -> ("error out"=w408:errorcluster)  [unwired: 1 in, 8 out]
          }
          event "Templates": Value Change {
            n175 = event-data() -> ("CtlRef"=w421:refnum<vi>, "NewVal"=w432:string)  [unwired: 1 out]
            n176 = control-ref of="This VI"() -> (w436:refnum<vi>)
            n177 = Unbundle By Name(w437) -> ("Class.Templates"=w424:refnum<class "FakedArray.lvclass">)
            n178 = call <resource>:"Defer_FP_Updates.vi"("Defer Panel Updates"=TRUE, "error in (no error)"=w434, "lv_icon.vi in"=w436) -> ("error out"=w426:errorcluster, "lv icon.vi out"=w431:refnum<vi>)  [unwired: 7 out]
            n179 = call-dynamic "SET_ScrollbarPosition.vi"("error in (no error)"=w426, "FakedArray.lvclass in"=w424) -> ("error out"=w428:errorcluster, "FakedArray.lvclass out"=w427:refnum<class "FakedArray.lvclass">)  [unwired: 1 in, 7 out]
            n180 = local write "Filter templates by keyword"("") -> ()
            n181 = call <resource>:"ResetColor.vi"("error in (no error)"=w428, "FakedArray in"=w427) -> ("error out"=w429:errorcluster, "FakedArray out"=w430:refnum<class "FakedArray.lvclass">)  [unwired: 8 out]
            n182 = call-dynamic "UpdateVisibleData.vi"("Templates tree"=w421, "error in (no error)"=w429, "Tag"=w432, "FakedArray in"=w430) -> ("error out"=w425:errorcluster, "FakedArray out"=w423:refnum<class "FakedArray.lvclass">)  [unwired: 1 in, 5 out]
            n183 = Bundle By Name(cluster=w437, "Class.Templates"=w423) -> (w422:T26)
            n184 = call <resource>:"Defer_FP_Updates.vi"("error in (no error)"=w425, "lv_icon.vi in"=w431) -> ("error out"=w433:errorcluster)  [unwired: 1 in, 8 out]
          }
          event "Templates": Mouse Down {
            n185 = event-data() -> ("CtlRef"=w442:refnum<vi>, "Coords"=w444:T29)  [unwired: 1 out]
            n186 = call <resource>:"Mouse Down_Tree.vi"("Tree"=w442, "error in (no error)"=w443, "Coords"=w444) -> ("error out"=w441:errorcluster)  [unwired: 8 out]
            n187 = call <resource>:"Escape.vi"("error in"=w441, "Data in"=w439) -> ("error out"=w440:errorcluster, "Data out"=w438:T26)  [unwired: 1 in, 7 out]
          }
          event Value Change {
            n188 = event-data() -> ("OldVal.Opacity"=w449:u8, "NewVal.Opacity"=w450:u8, "NewVal"=w454:T14)  [unwired: 1 out]
            n189 = Not Equal?(x=w449, y=w450) -> (x != y?=w448:bool)
            n190 = call <resource>:"Value Change_Top or Bottom Layer.vi"("Type"=enum16{"Template Layer", "Text Layer"}."Template Layer", "error in (no error)"=w456, "Data"=w454, "Data in"=w447) -> ("error out"=w452:errorcluster, "Data out"=w446:T26)  [unwired: 6 out]
            n191 = case shown="False" w448 {
              tunnel: w452 -> [w458 w462]
              tunnel: [w458 w461] -> w451
              tunnel: w446 -> [w457 w460]
              tunnel: [w457 w459] -> w445
              frame False {
              }
              frame True {
                n192 = call <resource>:"Reset layer template selection.vi"("error in (no error)"=w462, "Data in"=w460) -> ("error out"=w461:errorcluster, "Data out"=w459:T26)  [unwired: 1 in, 7 out]
              }
            }
          }
          event Mouse Down {
            n193 = event-data() -> ("CtlRef"=w468:refnum<vi>, "Button"=w464:u16)  [unwired: 1 out]
            n194 = case shown="1, 2" w464 {
              tunnel: w469 -> [w471 w478]
              tunnel: w468 -> [_ w482]
              tunnel: [w471 w476] -> w467
              tunnel: w465 -> [w470 w473]
              tunnel: [w470 w472] -> w463
              frame 0, Default {
              }
              frame 1, 2 {
                n195 = control-ref of="This VI"() -> (w481:refnum<vi>)
                n196 = call <resource>:"Defer_FP_Updates.vi"("Defer Panel Updates"=TRUE, "error in (no error)"=w478, "lv_icon.vi in"=w481) -> ("error out"=w479:errorcluster, "lv icon.vi out"=w474:refnum<vi>)  [unwired: 7 out]
                n197 = call <resource>:"Template_MouseDown.vi"("Add to Undo?"=TRUE, "error in"=w479, "CtlRef"=w482, "Data in"=w473) -> ("error out"=w477:errorcluster, "Data out"=w472:T26)  [unwired: 1 in, 5 out]
                n198 = call <resource>:"Defer_FP_Updates.vi"("error in (no error)"=w477, "lv_icon.vi in"=w474) -> ("error out"=w476:errorcluster)  [unwired: 1 in, 8 out]
              }
            }
          }
          event Value Change {
            n199 = event-data() -> ("NewVal"=w493:variant)  [unwired: 1 out]
            n200 = control-ref of="This VI"() -> (w490:refnum<vi>)
            n201 = call <resource>:"Defer_FP_Updates.vi"("Defer Panel Updates"=TRUE, "error in (no error)"=w491, "lv_icon.vi in"=w490) -> ("error out"=w492:errorcluster, "lv icon.vi out"=w485:refnum<vi>)  [unwired: 7 out]
            n202 = call <resource>:"Mouse Down_Templates.vi"("Tag"="Templates", "error in"=w492, "NewVal"=w493, "Data in"=w484) -> ("error out"=w487:errorcluster, "Data out"=w483:T26)  [unwired: 1 in, 5 out]
            n203 = call <resource>:"Defer_FP_Updates.vi"("error in (no error)"=w487, "lv_icon.vi in"=w485) -> ("error out"=w488:errorcluster)  [unwired: 1 in, 8 out]
          }
          event "Filter templates by keyword": Value Change {
            n204 = event-data() -> ("NewVal"=w513:string)  [unwired: 1 out]
            n205 = Unbundle By Name(w501) -> ("Ref.Templates tree"=w499:refnum<vi>, "Class.Templates"=w502:refnum<class "FakedArray.lvclass">)
            n206 = control-ref of="This VI"() -> (w512:refnum<vi>)
            n207 = call <resource>:"Defer_FP_Updates.vi"("Defer Panel Updates"=TRUE, "error in (no error)"=w510, "lv_icon.vi in"=w512) -> ("error out"=w504:errorcluster, "lv icon.vi out"=w509:refnum<vi>)  [unwired: 7 out]
            n208 = call-dynamic "SET_ScrollbarPosition.vi"("error in (no error)"=w504, "FakedArray.lvclass in"=w502) -> ("error out"=w505:errorcluster, "FakedArray.lvclass out"=w506:refnum<class "FakedArray.lvclass">)  [unwired: 1 in, 7 out]
            n209 = call <resource>:"ResetColor.vi"("error in (no error)"=w505, "FakedArray in"=w506) -> ("error out"=w507:errorcluster, "FakedArray out"=w508:refnum<class "FakedArray.lvclass">)  [unwired: 8 out]
            n210 = call-dynamic "UpdateVisibleData.vi"("Templates tree"=w499, "error in (no error)"=w507, "Keyword"=w513, "FakedArray in"=w508) -> ("error out"=w503:errorcluster, "FakedArray out"=w500:refnum<class "FakedArray.lvclass">)  [unwired: 1 in, 5 out]
            n211 = Bundle By Name(cluster=w501, "Class.Templates"=w500) -> (w495:T26)
            n212 = call <resource>:"Defer_FP_Updates.vi"("error in (no error)"=w503, "lv_icon.vi in"=w509) -> ("error out"=w497:errorcluster)  [unwired: 1 in, 8 out]
            n213 = call <resource>:"Add Data to History.vi"("Add to Undo?"=TRUE, "error in"=w497, "Data in"=w495) -> ("error out"=w496:errorcluster, "Data out"=w494:T26)  [unwired: 7 out]
          }
          event "Filter templates by keyword": Mouse Down {
            # "If a mouse down event should\nselect the entered text, enable this case"
            n214 = event-data() -> ("CtlRef"=w523:refnum<vi>)  [unwired: 1 out]
            n215 = disable-structure shown="Enabled" {
              disable-tunnel: w523 -> [w528 _]
              disable-tunnel: w522 -> [w526 w529]
              disable-tunnel: [w524 w529] -> w521
              frame Disabled {
                n216 = property class="Str"(reference=w528, error in=w526, "Text.Selection Start"=u32 0 ("Text.Selection:Start"), "Text.Selection End"=-1 ("Text.Selection:End")) -> (error out=w524:errorcluster)  [unwired: 1 out]
              }
              frame Enabled {
              }
            }
            n217 = call <resource>:"Finalize Text.vi"("error in (no error)"=w521, "Data in"=w519) -> ("error out"=w520:errorcluster, "Data out"=w518:T26)  [unwired: 8 out]
            n218 = call <resource>:"DeselectLayer.vi"("error in (no error)"=w520, "Data in"=w518) -> ("error out"=w517:errorcluster, "Data out"=w516:T26)  [unwired: 8 out]
            n219 = call <resource>:"Escape.vi"("error in"=w517, "Data in"=w516) -> ("error out"=w514:errorcluster, "Data out"=w515:T26)  [unwired: 1 in, 7 out]
          }
          event Value Change {
            n220 = event-data() -> ()  [unwired: 2 out]
            n221 = Unbundle By Name(w532) -> ("Ref.TemplateLoadAnimation"=w530:refnum<vi>, "Ref.refreshTemplates"=w531:refnum<vi>)
            n222 = call <resource>:"Launch Dynamically Load Graphics.vi"("User events"=w533, "Path"=Pathes."Icon Templates", "error in (no error)"=w535, "button ref"=w531, "animatedDecoration ref"=w530) -> ("error out"=w534:errorcluster)  [unwired: 1 in, 5 out]
          }
          event Mouse Down {
            n223 = event-data() -> ("CtlRef"=w541:refnum<vi>)  [unwired: 1 out]
            n224 = property class="CmbBox (strict)"(reference=w541, error in=w540, "Text.Selection Start"=u32 0 ("Text.Selection:Start"), "Text.Selection End"=u32 1000 ("Text.Selection:End")) -> (error out=w539:errorcluster)  [unwired: 1 out]
          }
          event Mouse Down {
            n225 = event-data() -> ()  [unwired: 2 out]
            n226 = call <resource>:"Escape.vi"("error in"=w544, "Data in"=w546) -> ("error out"=w543:errorcluster, "Data out"=w545:T26)  [unwired: 1 in, 7 out]
          }
          event Mouse Down {
            n227 = event-data() -> ()  [unwired: 2 out]
            n228 = call <resource>:"MouseDown_Body Text.vi"("error in"=w551, "Data in"=w548) -> ("error out"=w550:errorcluster, "Data out"=w547:T26)  [unwired: 8 out]
          }
          event Value Change {
            # "Body Text Value Change event is fired programmatically during initialization so first call of this event is guaranteed to be a case we do not want to update the undo/redo information."
            n229 = event-data() -> ("OldVal"=w560:T7, "NewVal"=w559:T7, "OldVal.Body Text Spec.Alignment"=w564:T9)  [unwired: 1 out]
            n230 = Unbundle By Name(w560) -> ("Body Text Spec.Font"=w558:T8)
            n231 = Unbundle By Name(w559) -> ("Body Text Spec.Font"=w557:T8)
            n232 = local read "Tab Control"() -> (w555:T3)
            n233 = Unbundle By Name(w559) -> ("Body Text Spec.Alignment"=w565:T9)
            n234 = First Call?() -> (First Call?: T/F=w572:bool)
            n235 = Equal?(x=w555, y=T3."Icon Text") -> (x = y?=w553:bool)
            n236 = Not(x=w572) -> (.not. x?=w571:bool)
            n237 = Not Equal?(x=w558, y=w557) -> (x != y?=w556:bool)
            n238 = call <resource>:"Value Change_Body Text.vi"("Layer Icon"="Icon Text", "Add to Undo?"=w571, "error in"=w573, "NewVal"=w559, "Data in"=w569) -> ("error out"=w567:errorcluster, "Data out"=w566:T26)  [unwired: 5 out]
            n239 = And(x=w553, y=w556) -> (x .and. y?=w552:bool)
            n240 = Not Equal?(x=w565, y=w564) -> (x != y?=w563:bool)
            n241 = case shown="False" w552 {
              frame False {
              }
              frame True {
                n242 = property on="Line 1 text" class="Str"("Key Focus"=TRUE) -> ()  [unwired: 2 in, 2 out]
              }
            }
            n243 = call <resource>:"Alignment Value Change.vi"("Set Focus?"=w563, "error in"=w567, "NewVal"=w565, "Data in"=w566) -> ("error out"=w561:errorcluster, "Data out"=w562:T26)  [unwired: 6 out]
          }
          event Value Change {
            n244 = event-data() -> ("OldVal.Opacity"=w580:u8, "NewVal.Opacity"=w579:u8, "NewVal"=w585:T14)  [unwired: 1 out]
            n245 = Not Equal?(x=w580, y=w579) -> (x != y?=w578:bool)
            n246 = call <resource>:"Value Change_Top or Bottom Layer.vi"("Type"=enum16{"Template Layer", "Text Layer"}."Text Layer", "error in (no error)"=w586, "Data"=w585, "Data in"=w577) -> ("error out"=w582:errorcluster, "Data out"=w576:T26)  [unwired: 6 out]
            n247 = case shown="True" w578 {
              tunnel: w582 -> [w588 w592]
              tunnel: [w588 w591] -> w581
              tunnel: w576 -> [w587 w590]
              tunnel: [w587 w589] -> w575
              frame False {
              }
              frame True {
                n248 = call <resource>:"Reset layer template selection.vi"("error in (no error)"=w592, "Data in"=w590) -> ("error out"=w591:errorcluster, "Data out"=w589:T26)  [unwired: 1 in, 7 out]
              }
            }
          }
          event Value Change {
            n249 = event-data() -> ("NewVal"=w603:variant)  [unwired: 1 out]
            n250 = control-ref of="This VI"() -> (w600:refnum<vi>)
            n251 = call <resource>:"Defer_FP_Updates.vi"("Defer Panel Updates"=TRUE, "error in (no error)"=w599, "lv_icon.vi in"=w600) -> ("error out"=w598:errorcluster, "lv icon.vi out"=w595:refnum<vi>)  [unwired: 7 out]
            n252 = Variant To Data(error in=w598, type=0, Variant=w603) -> (data=w602:i32, error out=w604:errorcluster)
            n253 = call <resource>:"UpdateLayerView_ScrollbarChanged.vi"("error in"=w604, "Scrollbar Position"=w602, "Data in"=w594) -> ("error out"=w597:errorcluster, "Data out"=w593:T26)  [unwired: 7 out]
            n254 = call <resource>:"Defer_FP_Updates.vi"("error in (no error)"=w597, "lv_icon.vi in"=w595) -> ("error out"=w596:errorcluster)  [unwired: 1 in, 8 out]
          }
          event Mouse Down {
            n255 = event-data() -> ("PlatMods.Shift"=w608:bool, "CtlRef"=w618:refnum<vi>, "PlatMods.Ctrl"=w617:bool)  [unwired: 1 out]
            n256 = control-ref of="This VI"() -> (w614:refnum<vi>)
            n257 = call <resource>:"Defer_FP_Updates.vi"("Defer Panel Updates"=TRUE, "error in (no error)"=w615, "lv_icon.vi in"=w614) -> ("error out"=w613:errorcluster, "lv icon.vi out"=w610:refnum<vi>)  [unwired: 7 out]
            n258 = call <resource>:"Mouse Down_User Layers.vi"("Shift"=w608, "error in"=w613, "Ctrl"=w617, "CtlRef"=w618, "Data in"=w607) -> ("error out"=w612:errorcluster, "Data out"=w606:T26)  [unwired: 5 out]
            n259 = call <resource>:"Defer_FP_Updates.vi"("error in (no error)"=w612, "lv_icon.vi in"=w610) -> ("error out"=w611:errorcluster)  [unwired: 1 in, 8 out]
          }
          event Mouse Down {
            n260 = event-data() -> ("Button"=w621:u16)  [unwired: 1 out]
            n261 = case shown="1" w621 {
              tunnel: w623 -> [w625 w629]
              tunnel: [w625 w628] -> w622
              tunnel: w620 -> [w624 w627]
              tunnel: [w624 w626] -> w619
              frame 0, Default {
              }
              frame 1 {
                # "Left click"
                n262 = call <resource>:"Reset layer template selection.vi"("error in (no error)"=w629, "Data in"=w627) -> ("error out"=w628:errorcluster, "Data out"=w626:T26)  [unwired: 1 in, 7 out]
              }
            }
          }
          event Value Change {
            # "We do not use the dynamic registerd event for Layer Clust.Value Change\nbecause it would be a huge effort to lock the front panel until this\nevent case has been completed."
            n263 = event-data() -> ("OldVal.Visibility?"=w631:bool, "CtlRef"=w645:refnum<vi>, "OldVal.LayerName"=w630:string)  [unwired: 1 out]
            n264 = control-ref of="This VI"() -> (w642:refnum<vi>)
            n265 = call <resource>:"Defer_FP_Updates.vi"("Defer Panel Updates"=TRUE, "error in (no error)"=w641, "lv_icon.vi in"=w642) -> ("error out"=w640:errorcluster, "lv icon.vi out"=w637:refnum<vi>)  [unwired: 7 out]
            n266 = call <resource>:"LayerCluster_ValueChange.vi"("Old Visibility?"=w631, "error in"=w640, "Old name"=w630, "CtlRef"=w645, "Data in"=w633) -> ("error out"=w639:errorcluster, "Data out"=w634:T26)  [unwired: 1 in, 4 out]
            n267 = call <resource>:"Defer_FP_Updates.vi"("Defer Panel Updates"=FALSE, "error in (no error)"=w639, "lv_icon.vi in"=w637) -> ("error out"=w636:errorcluster)  [unwired: 8 out]
            n268 = call <resource>:"Reset layer template selection.vi"("error in (no error)"=w636, "Data in"=w634) -> ("error out"=w635:errorcluster, "Data out"=w632:T26)  [unwired: 1 in, 7 out]
          }
          event Value Change {
            n269 = event-data() -> ()  [unwired: 2 out]
            n270 = control-ref of="This VI"() -> (w656:refnum<vi>)
            n271 = call <resource>:"Defer_FP_Updates.vi"("Defer Panel Updates"=TRUE, "error in (no error)"=w655, "lv_icon.vi in"=w656) -> ("error out"=w653:errorcluster, "lv icon.vi out"=w652:refnum<vi>)  [unwired: 7 out]
            n272 = call <resource>:"Add new Layer.vi"("error in"=w653, "Data in"=w657) -> ("error out"=w648:errorcluster, "Data out"=w650:T26)  [unwired: 8 out]
            n273 = call <resource>:"ViewLayer.vi"("Add to Undo?"=TRUE, "error in (no error)"=w648, "Data in"=w650) -> ("error out"=w647:errorcluster, "Data out"=w649:T26)  [unwired: 1 in, 6 out]
            n274 = call <resource>:"Defer_FP_Updates.vi"("error in (no error)"=w647, "lv_icon.vi in"=w652) -> ("error out"=w651:errorcluster)  [unwired: 1 in, 8 out]
          }
          event Mouse Leave; Mouse Up {
            n275 = event-data() -> ()  [unwired: 2 out]
            n276 = call <resource>:"Add Data to History.vi"("Add to Undo?"=TRUE, "error in"=w661, "Data in"=w658) -> ("error out"=w660:errorcluster, "Data out"=w659:T26)  [unwired: 7 out]
          }
          event Value Change {
            n277 = event-data() -> ()  [unwired: 2 out]
            n278 = control-ref of="This VI"() -> (w673:refnum<vi>)
            n279 = Unbundle By Name(w679) -> ("Class.Icon"=w678:refnum<class "Icon.lvclass">)
            n280 = call <resource>:"Defer_FP_Updates.vi"("Defer Panel Updates"=TRUE, "error in (no error)"=w672, "lv_icon.vi in"=w673) -> ("error out"=w671:errorcluster, "lv icon.vi out"=w670:refnum<vi>)  [unwired: 7 out]
            n281 = call-dynamic "GET_All User Layers.vi"("error in (no error)"=w671, "Icon.lvclass in"=w678) -> ("error out"=w685:errorcluster, "User Layer"=w681:refnum<class "Layer.lvclass">[], "Icon.lvclass out"=w680:refnum<class "Icon.lvclass">)  [unwired: 7 out]
            n282 = call <resource>:"Delete Selected Layers.vi"("error in"=w685, "All Layers in"=w681, "Data in"=w679) -> ("error out"=w684:errorcluster, "All Layers out"=w682:refnum<class "Layer.lvclass">[], "Data out"=w676:T26)
            n283 = call-dynamic "SET_UserLayers.vi"("error in (no error)"=w684, "Layers"=w682, "Icon.lvclass in"=w680) -> ("error out"=w683:errorcluster, "Icon.lvclass out"=w677:refnum<class "Icon.lvclass">)  [unwired: 7 in]
            n284 = Bundle By Name(cluster=w676, "Class.Icon"=w677) -> (w675:T26)
            n285 = call <resource>:"Reset layer template selection.vi"("error in (no error)"=w683, "Data in"=w675) -> ("error out"=w664:errorcluster, "Data out"=w666:T26)  [unwired: 1 in, 7 out]
            n286 = call <resource>:"ViewLayer.vi"("Add to Undo?"=TRUE, "error in (no error)"=w664, "Data in"=w666) -> ("error out"=w663:errorcluster, "Data out"=w665:T26)  [unwired: 2 in, 5 out]
            n287 = call <resource>:"Defer_FP_Updates.vi"("error in (no error)"=w663, "lv_icon.vi in"=w670) -> ("error out"=w669:errorcluster)  [unwired: 1 in, 8 out]
          }
          event Value Change {
            n288 = event-data() -> ()  [unwired: 2 out]
            n289 = control-ref of="This VI"() -> (w696:refnum<vi>)
            n290 = call <resource>:"Defer_FP_Updates.vi"("Defer Panel Updates"=TRUE, "error in (no error)"=w695, "lv_icon.vi in"=w696) -> ("error out"=w694:errorcluster, "lv icon.vi out"=w693:refnum<vi>)  [unwired: 7 out]
            n291 = call <resource>:"MoveLayers.vi"("error in"=w694, "Arrow Up"="Move Up", "Data in"=w690) -> ("error out"=w686:errorcluster, "Data out"=w689:T26)  [unwired: 7 out]
            n292 = stacked-sequence {
              tunnel: [w699] -> w687
              tunnel: w686 -> [w699]
              frame #0 {
                w700 = FALSE ("Arrow Down")
                n293 = local write "Move Down"(w700) -> ()
                n294 = local write "Move Up"(w700) -> ()
              }
            }
            n295 = call <resource>:"Defer_FP_Updates.vi"("Defer Panel Updates"=FALSE, "error in (no error)"=w687, "lv_icon.vi in"=w693) -> ("error out"=w692:errorcluster)  [unwired: 8 out]
          }
          event User Event {
            # "This is an initialization event for the glyphs."
            n296 = event-data() -> ("Glyphs"=w715:string)  [unwired: 1 out]
            n297 = Unbundle By Name(w703) -> ("Ref.GlyphLoadAnimation"=w702:refnum<vi>, "Ref.refreshGlyphs"=w701:refnum<vi>)
            n298 = Unflatten From String(type=T32[] [], binary string=w715, error in (no error)=w713) -> (value=w710:T32[], error out=w712:errorcluster)  [unwired: 3 out]
            n299 = call <resource>:"Populate Graphics.vi"("error in"=w712, "Glyphs []"=w710, "Data in"=w703) -> ("error out"=w711:errorcluster, "Data out"=w707:T26)  [unwired: 7 out]
            n300 = call <resource>:"Write Glyphs to  File.vi"("File Name"="Glyphs.bin", "Path"=Pathes."Glyphs", "error in (no error)"=w711, "Graphics []"=w710) -> ("error out"=w706:errorcluster)  [unwired: 7 out]
            n301 = call <resource>:"ChangeRefreshGraphicsState.vi"("error in (no error)"=w706, "refreshing?"=FALSE, "button ref"=w701, "animatedDecoration ref"=w702) -> ("error out"=w705:errorcluster)  [unwired: 7 in]
          }
          event "Glyphs": Mouse Down {
            n302 = event-data() -> ("CtlRef"=w717:refnum<vi>, "Coords"=w722:T29)  [unwired: 1 out]
            n303 = local write "Filter glyphs by keyword"("") -> ()
            n304 = call <resource>:"Mouse Down_Tree.vi"("Tree"=w717, "error in (no error)"=w723, "Coords"=w722) -> ("error out"=w721:errorcluster)  [unwired: 8 out]
            n305 = call <resource>:"Escape.vi"("error in"=w721, "Data in"=w719) -> ("error out"=w720:errorcluster, "Data out"=w718:T26)  [unwired: 1 in, 7 out]
          }
          event "Glyphs": Value Change {
            n306 = event-data() -> ("NewVal"=w731:string)  [unwired: 1 out]
            n307 = Unbundle By Name(w727) -> ("Class.Glyph"=w728:refnum<class "Glyph.lvclass">, "Ref.DNL_Glyphs []"=w724:refnum<vi>)
            n308 = call <resource>:"FilterGlyphs.vi"("error in (no error)"=w729, "DNL_Glyphs []"=w724, "Tag"=w731, "Glyph in"=w728) -> ("error out"=w730:errorcluster, "Glyph out"=w726:refnum<class "Glyph.lvclass">)  [unwired: 6 out]
            n309 = Bundle By Name(cluster=w727, "Class.Glyph"=w726) -> (w725:T26)
          }
          event "Filter glyphs by keyword": Mouse Down {
            # "If a mouse down event should\nselect the entered text, enable this case"
            n310 = event-data() -> ("CtlRef"=w740:refnum<vi>)  [unwired: 1 out]
            n311 = disable-structure shown="Disabled" {
              disable-tunnel: w741 -> [w744 w747]
              disable-tunnel: w740 -> [w743 _]
              disable-tunnel: [w742 w747] -> w739
              frame Disabled {
                n312 = property class="Str"(reference=w743, error in=w744, "Text.Selection Start"=u32 0 ("Text.Selection:Start"), "Text.Selection End"=-1 ("Text.Selection:End")) -> (error out=w742:errorcluster)  [unwired: 1 out]
              }
              frame Enabled {
              }
            }
            n313 = call <resource>:"Finalize Text.vi"("error in (no error)"=w739, "Data in"=w737) -> ("error out"=w738:errorcluster, "Data out"=w736:T26)  [unwired: 8 out]
            n314 = call <resource>:"DeselectLayer.vi"("error in (no error)"=w738, "Data in"=w736) -> ("error out"=w735:errorcluster, "Data out"=w734:T26)  [unwired: 8 out]
            n315 = call <resource>:"Escape.vi"("error in"=w735, "Data in"=w734) -> ("error out"=w732:errorcluster, "Data out"=w733:T26)  [unwired: 1 in, 7 out]
          }
          event "Filter glyphs by keyword": Value Change {
            n316 = event-data() -> ("NewVal"=w761:string)  [unwired: 1 out]
            n317 = Unbundle By Name(w756) -> ("Class.Glyph"=w757:refnum<class "Glyph.lvclass">, "Ref.DNL_Glyphs []"=w754:refnum<vi>, "Ref.Glyphs tree"=w753:refnum<vi>)
            n318 = First Call?() -> (First Call?: T/F=w759:bool)
            n319 = Not(x=w759) -> (.not. x?=w760:bool)
            n320 = call <resource>:"SearchGlyphs.vi"("Glyphs tree"=w753, "DNL_Glyphs []"=w754, "Reset position? (F)"=w760, "error in (no error)"=w758, "Keyword"=w761, "Glyph in"=w757) -> ("error out"=w752:errorcluster, "Glyph out"=w755:refnum<class "Glyph.lvclass">)  [unwired: 4 out]
            n321 = Bundle By Name(cluster=w756, "Class.Glyph"=w755) -> (w749:T26)
            n322 = call <resource>:"Add Data to History.vi"("Add to Undo?"=TRUE, "error in"=w752, "Data in"=w749) -> ("error out"=w751:errorcluster, "Data out"=w750:T26)  [unwired: 7 out]
          }
          event "Glyphs []": Mouse Down {
            n323 = event-data() -> ("Button"=w770:u16, "Mods.Double Click"=w771:bool, "CtlRef"=w773:refnum<vi>, "Coords"=w774:T29)  [unwired: 1 out]
            n324 = case shown="1" w770 {
              tunnel: w774 -> [_ w783]
              tunnel: w773 -> [_ w782]
              tunnel: [w776 w781] -> w767
              tunnel: w772 -> [w776 w780]
              tunnel: w771 -> [_ w779]
              tunnel: w765 -> [w775 w778]
              tunnel: [w775 w777] -> w763
              frame 0, Default {
              }
              frame 1 {
                # "Left click"
                n325 = call <resource>:"Mouse Down_Glyphs.vi"("Double Click"=w779, "Coords"=w783, "error in"=w780, "CtlRef"=w782, "Data in"=w778) -> ("error out"=w781:errorcluster, "Data out"=w777:T26)  [unwired: 1 in, 4 out]
              }
            }
            n326 = call <resource>:"Reset layer template selection.vi"("error in (no error)"=w767, "Data in"=w763) -> ("error out"=w766:errorcluster, "Data out"=w764:T26)  [unwired: 1 in, 7 out]
            n327 = call <resource>:"Update glyph path string.vi"("error in (no error)"=w766, "Data in"=w764) -> ("error out"=w768:errorcluster, "Data out"=w762:T26)  [unwired: 1 in, 7 out]
          }
          event Value Change {
            n328 = event-data() -> ()  [unwired: 2 out]
            n329 = Unbundle By Name(w786) -> ("Ref.GlyphLoadAnimation"=w784:refnum<vi>, "Ref.refreshGlyphs"=w785:refnum<vi>)
            n330 = call <resource>:"Launch Dynamically Load Graphics.vi"("User events"=w787, "Path"=Pathes."Glyphs", "error in (no error)"=w789, "button ref"=w785, "animatedDecoration ref"=w784) -> ("error out"=w788:errorcluster)  [unwired: 1 in, 5 out]
          }
          event "Help": Value Change {
            n331 = event-data() -> ()  [unwired: 2 out]
            n332 = control-ref of="This VI"() -> (w793:refnum<vi>)
            n333 = property class="VI"(reference=w793) -> (error out=w791:errorcluster, "Help.URL"=w792:string)  [unwired: 1 in, 1 out]
            n334 = call <resource>:"IE_Open Help Link.vi"("error in (no error)"=w791, "Help.URL"=w792) -> ()  [unwired: 9 in, 1 out]
          }
          event "Glyphs", "Templates": Item Close; "Glyphs", "Templates": event #0x1e {
            n335 = event-data() -> ("CtlRef"=w796:refnum<vi>)  [unwired: 1 out]
            n336 = call <resource>:"DealWithScrollbars.vi"("error in (no error)"=w798, "Tree"=w796) -> ("error out"=w797:errorcluster)  [unwired: 9 in]
          }
        }
        n337 = case shown="True" w146 {
          tunnel: [_ w162] -> w149
          tunnel: w148 -> [w159 w165]
          tunnel: [w159 w164] -> w147
          tunnel: "Tools" -> [_ w163]
          tunnel: w157 -> [w158 w161]
          tunnel: [w158 w160] -> w156
          frame False {
          }
          frame True {
            n338 = call <resource>:"DrawIcon.vi"("Tools"=w163, "error in (no error)"=w165, "Data in"=w161) -> ("error out"=w164:errorcluster, "Icon"=w162:picture, "Data out"=w160:T26, "RGB"=→"RGB":string, "XYL"=→"XYZ":string)  [unwired: 2 in, 2 out]
            "Icon" <- w162
            "Preview" <- w162
          }
        }
        n339 = Or(x=w148, y=w153) -> (x .or. y?=w152:bool)
      }
      n340 = call <resource>:"Buffer for lossless tracking.vi"("Ref Cluster"=w127, "User events"=w110, "error in (no error)"=w131, "Buffer"=w130) -> ()  [unwired: 8 out]
      n341 = call <resource>:"Extract LV Icon Data.vi"("error in (no error)"=w121, "LabVIEW Icon in (original)"=w119, "Data in"=w123) -> ("error out"=w120:errorcluster, "LabVIEW Icon out"=w122:string, "Data out"=w118:T26)  [unwired: 6 in]
      n342 = call <vilib>:"Get Image Data.vi"("Pic In"=w138) -> ("image data out"=w126:T2)  [unwired: 2 in, 8 out]
      n343 = call <vilib>:"Get Image Data.vi"("depth (24)"=1 ("depth"), "Pic In"=w138) -> ("image data out"=w136:T2)  [unwired: 2 in, 7 out]
      n344 = call <resource>:"SetCursor.vi"("Radio Buttons"=Tools."Select", "Data in"=w118) -> ("Data out"=w117:T26)  [unwired: 8 in, 1 out]
      n345 = Unbundle By Name(w120) -> ("code"=w139:i32)
      n346 = flat-sequence {
        tunnel: w142 -> [w800]
        tunnel: w140 -> [w812]
        tunnel: w120 -> [w811]
        tunnel: w110 -> [w809]
        tunnel: w117 -> [w805]
        tunnel: w115 -> [w803]
        tunnel: [w803] -> w114
        tunnel: [w802] -> w113
        tunnel: [w801] -> w112
        tunnel: w111 -> [w801]
        tunnel: w114 -> [w818]
        tunnel: w113 -> [w817]
        tunnel: w112 -> [w815]
        frame #0 {
          n347 = Unbundle By Name(w809) -> ("Global stop?"=w808:refnum<user-event>, "Templates"=w807:refnum<user-event>, "Glyphs"=w806:refnum<user-event>)
          n348 = call <resource>:"Write INI Tokens and VI Tags.vi"("error in (no error)"=w811, "Data in"=w805) -> ("error out"=w804:errorcluster)  [unwired: 1 in, 8 out]
          n349 = Unregister For Events(event registration refnum=w800) -> ()  [unwired: 1 in, 1 out]
          n350 = flat-sequence {
            tunnel: w804 -> [_]
            tunnel: [w814] -> w802
            frame #0 {
              n351 = call <resource>:"Call Keep IE in Memory.vi"() -> ()  [unwired: 1 out]
            }
            frame #1 {
              n352 = property class="VI"() -> ("Front Panel.WinBounds"=w814:T36)  [unwired: 2 in, 2 out]
            }
          }
          n353 = Release Notifier(notifier=w812, force destroy? (F)=TRUE) -> ()  [unwired: 1 in, 3 out]
          n354 = Generate User Event(user event=w808, event data cluster=TRUE) -> ()  [unwired: 2 in, 2 out]
          n355 = Destroy User Event(user event=w807) -> ()  [unwired: 1 in, 1 out]
          n356 = Destroy User Event(user event=w806) -> ()  [unwired: 1 in, 1 out]
        }
        frame #1 {
          n357 = Equal?(x=w817, y=w818) -> (x = y?=w816:bool)
          n358 = case shown="False" w816 {
            tunnel: w817 -> [w826 _]
            tunnel: w815 -> [w819 _]
            frame False {
              # "Bounds changed...write new bounds\nto INI file"
              n359 = Unbundle(w826) -> ("Left"=w825:i16, "Top"=w824:i16, "Right"=w823:i16, "Bottom"=w822:i16)
              n360 = Format Into String(format string="%d,%d,%d,%d", w825, w824, w823, w822) -> (resulting string=w820:string)  [unwired: 2 in, 1 out]
              n361 = call-by-ref "?"("value"=w820, "key"=w819) -> ()  [unwired: 3 in, 7 out]
            }
            frame True {
              # "Bounds didn't change while window was\nopen...don't do anything"
            }
          }
        }
        frame #2 {
          n362 = invoke class="VI" method="FP.Close"() -> ()  [unwired: 3 in, 3 out]
        }
      }
      n363 = call-dynamic "GET_Notifier.vi"("error in (no error)"=w124, "Ants.lvclass in"=w128) -> ("error out"=w134:errorcluster, "Notifier"=w140:refnum<notifier>, "Ants.lvclass out"=w135:refnum<class "Ants.lvclass">)  [unwired: 7 out]
      n364 = call <resource>:"RunningAnts.vi"("error in (no error)"=w134, "Ants in"=w135) -> ()  [unwired: 10 out]
    }
    frame Error {
      n365 = Unbundle By Name(w828) -> ("code"=w829:i32)
      n366 = call <vilib>:"Simple Error Handler.vi"("error in (no error)"=w828) -> ()  [unwired: 4 in, 5 out]
    }
  }
  "BW icon out" <- w57
  "Error code out" <- w62
  "Color icon out" <- w39
  "LabVIEW Icon out" <- w36
